vi "Oxford-1820-Main_.vi"() -> ()   [LabVIEW 2016]
uses:
  <instrlib>/Mercury iXX/Public/Controls/Unit String.ctl
  <instrlib>/Mercury iXX/Public/Libraries/Temperature/Controls/Temperature Device (Read).ctl
  <instrlib>/Mercury iXX/Public/Controls/Manufacturing Data.ctl
  <instrlib>/Mercury iXX/Public/Libraries/Temperature/Controls/Temperature Sensor Type.ctl
  <instrlib>/Mercury iXX/Public/Libraries/Temperature/Controls/Excitation Cluster.ctl
  <instrlib>/Mercury iXX/Public/Libraries/Temperature/Controls/Excitation Type.ctl
  <instrlib>/Mercury iXX/Public/Libraries/Temperature/Controls/Calibration Cluster.ctl
  <instrlib>/Mercury iXX/Public/Libraries/Temperature/Controls/Calibration Interpolation.ctl
  <instrlib>/Mercury iXX/Public/Libraries/Temperature/Controls/Loop Cluster.ctl
  <instrlib>/Mercury iXX/Public/Libraries/Temperature/Controls/Temperature Signals Cluster.ctl
  <instrlib>/Mercury iXX/Public/Libraries/Heater/Controls/Heater Device (Read).ctl
  <instrlib>/Mercury iXX/Public/Libraries/Heater/Controls/Heater Signals Cluster.ctl
  <instrlib>/Mercury iXX/Public/Libraries/Level Meter/Controls/Level Meter (Read).ctl
  <instrlib>/Mercury iXX/Public/Libraries/Level Meter/Controls/Nitrogen Configuration.ctl
  <instrlib>/Mercury iXX/Public/Libraries/Level Meter/Controls/Frequency Configuration.ctl
  <instrlib>/Mercury iXX/Public/Libraries/Level Meter/Controls/Signals.ctl
  <instrlib>/Mercury iXX/Public/Libraries/Level Meter/Controls/Helium Configuration.ctl
  <instrlib>/Mercury iXX/Public/Libraries/Level Meter/Controls/Resistance Configuration.ctl
  <instrlib>/Mercury iXX/Public/Libraries/Level Meter/Controls/Pre-Pulse.ctl
  <instrlib>/Mercury iXX/Public/Libraries/Level Meter/Controls/Pulse.ctl
  <instrlib>/Mercury iXX/Public/Libraries/Auxiliary/Controls/AUX Device (Read).ctl
  <instrlib>/Mercury iXX/Public/Libraries/Auxiliary/Controls/AUX Signals (Read).ctl
  <instrlib>/Mercury iXX/Public/Libraries/Magnet/Controls/Device (Read).ctl
  <instrlib>/Mercury iXX/Public/Libraries/Magnet/Controls/Signals (Read).ctl
  <instrlib>/Mercury iXX/Public/Libraries/Magnet/Controls/Identifier.ctl
  <instrlib>/Mercury iXX/Public/Libraries/Pressure/Controls/Pressure Device (Read).ctl
  <instrlib>/Mercury iXX/Public/Libraries/Pressure/Controls/Pressure Sensor Type.ctl
  <instrlib>/Mercury iXX/Public/Libraries/Pressure/Controls/Calibration Cluster.ctl
  <instrlib>/Mercury iXX/Public/Libraries/Pressure/Controls/Calibration Interpolation.ctl
  <instrlib>/Mercury iXX/Public/Libraries/Pressure/Controls/Loop Cluster.ctl
  <instrlib>/Mercury iXX/Public/Libraries/Pressure/Controls/Pressure Signals Cluster.ctl
  <instrlib>/Mercury iXX/Mercury iXX.lvlib
  <instrlib>/Mercury iXX/Public/Controls/Comms Transport Layer.ctl
  <instrlib>/Mercury iXX/Public/Libraries/Pressure/Open/Open Pressure Device.vi
  <instrlib>/Mercury iXX/Public/Libraries/Pressure.lvlib
  <instrlib>/Mercury iXX/Public/Libraries/Pressure/Configuration/Read/Pressure Device (Read).vi
  <instrlib>/Mercury iXX/Public/Libraries/System/Read/Display Automatic Dimming (Read).vi
  <instrlib>/Mercury iXX/Public/Libraries/System.lvlib
  <instrlib>/Mercury iXX/Public/Libraries/System/Read/Display Automatic Dimming Time (Read).vi
  <instrlib>/Mercury iXX/Public/Libraries/System/Read/Display Brightness (Read).vi
  <instrlib>/Mercury iXX/Public/Libraries/System/Read/Mode (Read).vi
  <instrlib>/Mercury iXX/Public/Libraries/System/Read/Serial Number (Read).vi
  <instrlib>/Mercury iXX/Public/Libraries/System/Read/FVer (Read).vi
  <instrlib>/Mercury iXX/Public/Libraries/System/Read/HVer (Read).vi
  <instrlib>/Mercury iXX/Public/Libraries/System/Set/DateTime (Set).vi
  <instrlib>/Mercury iXX/Public/Libraries/Control Loop/Configuration/Read/Control Loop (Read).vi
  <instrlib>/Mercury iXX/Public/Libraries/Control Loop.lvlib
  <instrlib>/Mercury iXX/Public/Libraries/Temperature/Signals/Read/Temperature (Read).vi
  <instrlib>/Mercury iXX/Public/Libraries/Temperature.lvlib
  <instrlib>/Mercury iXX/Public/Libraries/Temperature/Configuration/Read/Calibration Cold Limit (Read).vi
  <instrlib>/Mercury iXX/Public/Libraries/Temperature/Configuration/Read/Calibration Hot Limit (Read).vi
  <instrlib>/Mercury iXX/Public/Libraries/Temperature/Configuration/Read/Excitation Type (Read).vi
  <instrlib>/Mercury iXX/Public/Libraries/Temperature/Configuration/Read/Temperature Sensor (Read).vi
  <instrlib>/Mercury iXX/Public/Libraries/Temperature/Configuration/Read/Temperature Device (Read).vi
  <instrlib>/Mercury iXX/Public/Libraries/Temperature/Configuration/Read/Nickname (Read).vi
  <instrlib>/Mercury iXX/Public/Libraries/Temperature/Configuration/Read/Excitation Magnitude (Read).vi
  <instrlib>/Mercury iXX/Public/Libraries/Temperature/Configuration/Read/Serial Number (Read).vi
  <instrlib>/Mercury iXX/Public/Libraries/System/Read/Catalogue (Read).vi
  <instrlib>/Mercury iXX/Public/Libraries/System/Read/Flash Space (Read).vi
  <instrlib>/Mercury iXX/Public/Libraries/System/Read/DateTime (Read).vi
  <instrlib>/Mercury iXX/Public/Libraries/System/Read/Time (Read).vi
  <instrlib>/Mercury iXX/Public/Libraries/System/Read/Date (Read).vi
  <instrlib>/Mercury iXX/Public/Libraries/System/Open/Open System.vi
  <instrlib>/Mercury iXX/Public/Libraries/Temperature/Open/Open Temperature Device.vi
  <instrlib>/Mercury iXX/Public/Libraries/Auxiliary/Open/Open Auxiliary Device.vi
  <instrlib>/Mercury iXX/Public/Libraries/Auxiliary.lvlib
  <instrlib>/Mercury iXX/Public/Libraries/Auxiliary/Signals/Read/Percent Open (Read).vi
  <instrlib>/Mercury iXX/Public/Libraries/Magnet/Open/Open Magnet Device.vi
  <instrlib>/Mercury iXX/Public/Libraries/Magnet.lvlib
  <instrlib>/Mercury iXX/Public/Libraries/Magnet/Configuration/Read/PSU Action Status (Read).vi
  <instrlib>/Mercury iXX/Public/Libraries/Magnet/Configuration/Read/Magnet Device (Read).vi
  <instrlib>/Mercury iXX/Public/Libraries/Temperature/Signals/Read/Voltage (Read).vi
  <instrlib>/Mercury iXX/Private/Controls/Query Dynamic Reference.ctl
  <instrlib>/Mercury iXX/Public/Controls/Mercury Reference.ctl
  <instrlib>/Mercury iXX/Public/Libraries/Level Meter/Open/Open Level Meter Device.vi
  <instrlib>/Mercury iXX/Public/Libraries/Level Meter.lvlib
  <instrlib>/Mercury iXX/Public/Libraries/Level Meter/Signals/Read/Probe Level Nitrogen (Read).vi
  <instrlib>/Mercury iXX/Public/Libraries/Level Meter/Signals/Read/Probe Level Helium (Read).vi
  <instrlib>/Mercury iXX/Public/Libraries/Magnet/Signals/Read/Switch Heater Status (Read).vi
  <instrlib>/Mercury iXX/Public/Libraries/Magnet/Signals/Read/Current (Read).vi
  <instrlib>/Mercury iXX/Public/Libraries/Magnet/Configuration/Set/PSU Action Status (Set).vi
  <instrlib>/Mercury iXX/Public/Libraries/Magnet/Controls/PSU Actions.ctl
  SMOs/Instrument.Oxford1820/Instrument.Oxford1820.lvclass
  <instrlib>/Mercury iXX/Public/Controls/ISOBus Address.ctl
  <instrlib>/Mercury iXX/Public/Libraries/Lambda/Configuration/Set/Lambda Percentage Flow (Set).vi
  <instrlib>/Mercury iXX/Public/Libraries/Lambda.lvlib
  <instrlib>/Mercury iXX/Public/Libraries/Lambda/Open/Open Lambda Device.vi
  <instrlib>/Mercury iXX/Public/Controls/Response String.ctl
  <instrlib>/Mercury iXX/Public/Libraries/Temperature/Signals/Read/Resistance (Read).vi
  <instrlib>/Mercury iXX/Public/Libraries/Magnet/Controls/Switch Heater.ctl
  <instrlib>/Mercury iXX/Public/Libraries/Heater/Configuration/Read/Serial Number (Read).vi
  <instrlib>/Mercury iXX/Public/Libraries/Heater.lvlib
  <instrlib>/Mercury iXX/Public/Libraries/Pressure/Configuration/Read/Nickname (Read).vi
  <instrlib>/Mercury iXX/Public/Libraries/Level Meter/Configuration/Set/Pulse Slow-Fast (Set).vi
  <instrlib>/Mercury iXX/Public/Libraries/Magnet/Signals/Set/Target Field Rate (Set).vi
  <instrlib>/Mercury iXX/Public/Libraries/Auxiliary/Configuration/Read/Stepper Speed (Read).vi
  <instrlib>/Mercury iXX/Public/Libraries/Heater/Configuration/Read/Nickname (Read).vi
  <instrlib>/Mercury iXX/Public/Libraries/Auxiliary/Signals/Read/Position (Read).vi
  <instrlib>/Mercury iXX/Public/Libraries/Pressure/Signals/Read/Current (Read).vi
  <instrlib>/Mercury iXX/Public/Libraries/Auxiliary/Configuration/Read/Temperature Error Voltage Sensitivity (Read).vi
  <instrlib>/Mercury iXX/Public/Libraries/Heater/Signals/Read/Voltage (Read).vi
  <instrlib>/Mercury iXX/Public/Libraries/Heater/Configuration/Read/Maximum Power (Read).vi
  <instrlib>/Mercury iXX/Public/Libraries/Auxiliary/Configuration/Read/Temperature Error Sensitivity (Read).vi
  <instrlib>/Mercury iXX/Public/Libraries/Auxiliary/Configuration/Read/Aux Device (Read).vi
  <instrlib>/Mercury iXX/Public/Libraries/Heater/Open/Open Heater Device.vi
  <instrlib>/Mercury iXX/Public/Libraries/Heater/Signals/Read/Current (Read).vi
  <userlib>/_OpenG.lib/error/error.llb/Filter Error Codes (Array)__ogtk.vi
  <instrlib>/Mercury iXX/Public/Libraries/Lambda/Configuration/Set/Lambda Flow Auto (Set).vi
  <instrlib>/Mercury iXX/Public/Libraries/Heater/Configuration/Read/Heater Device (Read).vi
  <instrlib>/Mercury iXX/Public/Libraries/Auxiliary/Configuration/Read/Valve Gearing (Read).vi
  <instrlib>/Mercury iXX/Public/Libraries/Auxiliary/Configuration/Read/Serial Number (Read).vi
  <instrlib>/Mercury iXX/Public/Libraries/Heater/Configuration/Read/Voltage Limit (Read).vi
  <instrlib>/Mercury iXX/Public/Libraries/Heater/Configuration/Read/Nominal Resistance (Read).vi
  <instrlib>/Mercury iXX/Public/Libraries/Pressure/Signals/Read/Voltage (Read).vi
  <instrlib>/Mercury iXX/Public/Libraries/Magnet/Signals/Set/Target Field (Set).vi
  <instrlib>/Mercury iXX/Public/Libraries/Magnet/Signals/Read/Persistant Current (Read).vi
  <instrlib>/Mercury iXX/Public/Libraries/Auxiliary/Configuration/Read/Minimum Gas Flow (Read).vi
  <instrlib>/Mercury iXX/Public/Libraries/Heater/Signals/Read/Power (Read).vi
  <instrlib>/Mercury iXX/Public/Libraries/Auxiliary/Configuration/Read/Gas Flow Scaling (Read).vi
  <instrlib>/Mercury iXX/Public/Libraries/Magnet/Signals/Set/Switch Heater Status (Set).vi
  <instrlib>/Mercury iXX/Public/Libraries/Level Meter/Configuration/Read/Nitrogen Freq at 100 (Read).vi
  <instrlib>/Mercury iXX/Public/Libraries/Magnet/Configuration/Read/Serial Number (Read).vi
  <instrlib>/Mercury iXX/Public/Libraries/Magnet/Signals/Read/Field (Read).vi
  <instrlib>/Mercury iXX/Public/Libraries/Level Meter/Configuration/Read/Helium Pulse Mag (Read).vi
  <instrlib>/Mercury iXX/Public/Libraries/Level Meter/Configuration/Read/Helium Probe Resistance (Read).vi
  <instrlib>/Mercury iXX/Public/Libraries/Magnet/Signals/Read/Voltage (Read).vi
  <instrlib>/Mercury iXX/Public/Libraries/Magnet/Configuration/Read/Current to Field Factor (Read).vi
  <instrlib>/Mercury iXX/Public/Libraries/Magnet/Signals/Read/Target Field (Read).vi
  <instrlib>/Mercury iXX/Public/Libraries/Magnet/Configuration/Read/Bipolar Output (Read).vi
  <instrlib>/Mercury iXX/Public/Libraries/Magnet/Configuration/Read/Current Limit (Read).vi
  <instrlib>/Mercury iXX/Public/Libraries/Magnet/Signals/Read/Persistant Field (Read).vi
  <instrlib>/Mercury iXX/Public/Libraries/Level Meter/Configuration/Read/Serial Number (Read).vi
  <instrlib>/Mercury iXX/Public/Libraries/Magnet/Signals/Read/Current Rate (Read).vi
  <instrlib>/Mercury iXX/Public/Libraries/Magnet/Signals/Read/Target Field Rate (Read).vi
  <instrlib>/Mercury iXX/Public/Libraries/Level Meter/Configuration/Read/Level Meter Device (Read).vi
  <instrlib>/Mercury iXX/Public/Libraries/Level Meter/Signals/Read/Probe Resistance Helium (Read).vi
  <instrlib>/Mercury iXX/Public/Libraries/Magnet/Configuration/Read/Output Configuration (Read).vi
  <instrlib>/Mercury iXX/Public/Libraries/Level Meter/Configuration/Read/Nitrogen Pulse Count Period (Read).vi
  <instrlib>/Mercury iXX/Public/Libraries/Magnet/Configuration/Read/Software Voltage Limit (Read).vi
  <instrlib>/Mercury iXX/Public/Libraries/Level Meter/Configuration/Read/Helium Pulse Duration (Read).vi
  <instrlib>/Mercury iXX/Public/Libraries/Level Meter/Signals/Read/Probe Count Nitrogen (Read).vi
  <instrlib>/Mercury iXX/Public/Libraries/Magnet/Configuration/Read/Switch Present (Read).vi
panel:
  in  "Tab Control 6":enum32{"Page 1", "Page 2"}(tab)
  in  "Tab Control 5":enum32{"Page 1", "Page 2"}(tab)
  in  "Open Needle Valve":bool
  in  "Close Needle Valve":bool
  in  "Lambda":bool
  out "LPF NV (%)":dbl format="%_6g"
  out "LPF Pressure":dbl format="%_5f mB"
  out "Magnet Field (T) 2":dbl(knob) caption="Voltage (V)" scale=-20.0..20.0
  out "Voltage (V) 2":dbl(knob)=-0.0003 caption="Voltage (V)" scale=-10.0..10.0
  out "Current (A)":dbl(knob)=0.0006 scale=-180.0..180.0
  in  "Tab Control 4":enum32{"Page 1", "Page 2"}(tab)
  out "N2 LEVEL":dbl=61.3025 format="%.0f %"
  out "He LVL Chart":dbl(slide)=52.0833 scale=0.0..100.0
  out "N2 LVL Chart":dbl(slide)=61.3025 scale=0.0..100.0
  out "He LEVEL 3":dbl=61.3025 format="%.0f %"
  in  "Fast/Slow Fill":bool
  in  "Tab Control 3":enum32{"Page 1", "Page 2"}(tab)
  out "Magnet T":dbl=3.8705 format="%_2f K"
  out "Magnet R":dbl=3.8705 format="%_3f ohms"
  out "LPF R":dbl=4.2075 format="%_3f ohms"
  out "Voltage (V)":dbl=-0.0003 format="%.5f"
  out "LPF T":dbl=4.2075 format="%_2f K"
  out "Current (A)":dbl=0.0006 format="%.5f"
  out "Magnet Status 2":string
  in  "Tab Control 2":enum32{"Page 1", "Page 2"}(tab)
  in  "Hold":bool
  in  "To Set":bool
  in  "Send to IPS":bool
  out "Power Supply Field (T)":dbl=0.0001 format="%#.5f"
  in  "Target Field (T) 2":dbl format="%#.5f"
  out "Target Field (T)":dbl format="%#.5f"
  in  "Target Rate (T/min)":dbl=0.1 format="%.5f"
  out "Target  Rate (T/min)":dbl=1.0 format="%.5f"
  out "Magnet Field (T)":dbl format="%.5f"
  out "He LEVEL":dbl=52.0833 format="%.0f %"
  in  "PS Heat":bool
  out "Switch Time":string="11:11:48"
  in  "To Zero":bool
  in  "Clamp":bool
  in  "Toolbar":enum32{"Page 1", "Page 2"}(tab)
  in  "Start 2":bool
  in  "Stop 2":bool
  in  "Window Minimize":bool
  out "ETA":string
  out "Magnet Status 3":string="Clamped"
  in  "Remote Mode":bool
  out "Sentinel":bool=TRUE
  in  "Window Maximize":bool
  out "SWITCH HEATER":bool
  out "LPF ON":timestamp
  in  "Tab Control":T1(tab)
  in  "Mercury Functions":T2(tab)=enum."Temperature"
  out "time stamp":timestamp=timestamp(3543841780 s since 1904-01-01)
  out "Free Space":i32=166384 caption="Free Space (KB)"
  out "Set Date Response":string="VALID"
  out "String":string="NORM" caption="User Mode"
  out "Date":string="2016:04:18"
  out "Time":string="11:29:40"
  out "Hardware Version":string="65"
  out "Firmware Version":string="2.2.6.20"
  out "Serial Number":string="154650110"
  out "ITC Devices":string[](array[string])=["DB4.G1:AUX", "DB8.P1:PRES", "MB0.H1:HTR", "MB1.T1:TEMP"]
  out "S/W Version(s)":string[](array[string])=["2.2.6.20\n"]
  out "Serial Number(s)":string[](array[string])=["154650110"]
  out "# of Instruments":i32=1
  out "Automatic Dimming":string="OFF"
  out "Dimming Time":string="5"
  out "Display Brightness":string="100"
  in  "ITC IP Address":string="130.49.180.101"
  out "Excitation Magnitude":dbl=5.0
  out "Sensor Type":string="NTC"
  out "Excitation Type":string="UNIP"
  out "Hot Limit":dbl=1000.0
  out "H Unit":T3="K"
  out "Cold Limit":dbl=1000.0
  out "C Unit":T3="K"
  out "Unit":T3
  out "Voltage":dbl=0.005
  out "V Unit":T3="V"
  out "Temperature":dbl=4.2075
  out "T Unit":T3="K"
  out "Temperature Device Settings":T4={"Manufacturing"={"Hardware Version"="65", "Firmware Version"="2.2", "Serial Number"="154650110"}, "Temperature Sensor Type"="NTC", "Excitation"={"Excitation Type"="UNIP", "Magnitude"="5.00"}, "Calibration"={"Filename"="59543_iTC-lambda.dat", "Interpolation"="LIN", "Scaling Factor"="1", "Offset Factor"="0", "Hot Limit"="1000.00K", "Cold Limit"="1000.00K", "Last Calibration"="", "Reference"="Internal"}, "Control Loop"={"Heater"="", "Auxiliary"="", "Heater Auto"="", "Percentage Heat"="", "Temperature Set Point"="", "PID Auto (from file)"="", "P Value"="", "I Value"="", "D Value"="", "Auto PID Table Filename"="", "Flow Auto"="", "Target Heater Table"="", "Sweep mode"="", "Sweep Table Filename"="", "Percentage Flow"=""}, "Temperature Signals"={"Voltage"="5.0000mV", "Current"="3.9694µA", "Power"="0.0199µW", "Resistance"="1259.6510R", "Temperature"="4.2075K", "Sensitivity"="299.3801R/K", "Reference"="N/A"}, "Nickname"="Mag_AB_MB1", "Status"="0"}
  out "Temp S/N":string="154650110"
  out "T Nickname":string="Mag_AB_MB1"
  out "T Loop Details":T11
  out "Heater Device Settings":T13={"Manufacturing"={"Hardware Version"="65", "Firmware Version"="2.3", "Serial Number"="154650110"}, "Nickname"="MB0.H1", "Voltage Limit"="1", "Nominal Resistance"="10", "Maximum Power"="0.1000", "Heater Signals"={"Voltage"="0.0507V", "Current"="-0.0000A", "Power"="0.0000W"}, "Status"="2"}
  out "Htr C Unit":T3="A"
  out "Htr P Unit":T3="W"
  out "Htr V Unit":T3="V"
  out "Htr Current":dbl=-0.0
  out "Htr Power":dbl
  out "Htr Voltage":dbl=0.0507
  out "Power Unit":T3
  out "Volt Unit":T3
  out "Res Unit":T3
  out "Maximum Power":dbl=0.1
  out "Htr Resistance":dbl=10.0
  out "Htr Voltage Limit":dbl=1.0
  out "Htr S/N":string="154650110"
  out "Htr Nickname":string="MB0.H1"
  out "Pressure Device":T15={"Manufacturing"={"Hardware Version"="3", "Firmware Version"="1.10", "Serial Number"="151150091"}, "Temperature Sensor Type"="RAT", "Calibration"={"Filename"="Lambda pressure control_10V ratiometric.dat", "Interpolation"="LIN", "Scaling Factor"="1", "Offset Factor"="-0.0004", "High Limit"="1000.00K", "Low Limit"="1000.00K", "Last Calibration"=""}, "Control Loop"={"Heater"="None", "Auxiliary"="None", "Heater Auto"="", "Percentage Heat"="", "Pressure Set Point"="", "PID Auto (from file)"="", "P Value"="", "I Value"="", "D Value"="1.0", "Auto PID Table Filename"="", "Flow Auto"="", "Target Heater Table"="", "Sweep mode"="", "Sweep Table Filename"="", "Percentage Flow"=""}, "Pressure Signals"={"Voltage"="-0.0822mV", "Current"="-0.0000A", "Power"="0.0000W", "Pressure"="0.0000mB"}, "Nickname"="Lam_P_DB8", "Status"="0"}
  out "Nickname":string="Lam_P_DB8"
  out "Current":dbl=-0.0
  out "Voltage":dbl=-8.219999999999999e-05
  out "Auxiliary Device Details":T21={"Manufacturing"={"Hardware Version"="65", "Firmware Version"="3.1", "Serial Number"="154650084"}, "Min Flow"=0.0, "Scaling Factor"=50.0, "Temp Err"=9.0, "Temp V Err"=11.0, "Gear"=2, "Speed"=2, "Signals"={"Position"=0.0, "% Open"=0.0, "I0"="ON", "I1"="OFF", "I2"="OFF", "I3"="OFF", "O0"="OFF", "O1"="OFF", "O2"="OFF", "O3"="OFF"}, "Nickname"="DB4.G1", "Status"="0"} {"Signals"."% Open" min=0.0 max=100.0 step=0.1 format="%.4f"; "Signals"."Position" max=20.0 step=1.0 format="%.4f"; "Speed" max=7 step=1; "Gear" max=7 step=1; "Temp V Err" min=0.0 max=20.0 step=0.1; "Temp Err" min=0.0 max=20.0 step=0.1; "Scaling Factor" min=0.0 max=99.0 step=0.1; "Min Flow" min=0.0 max=20.0 step=0.1}
  out "Aux S/N":string="154650084"
  out "Min Flow":dbl caption="Minimum Gas Flow" format="%#.1f"
  out "Scaling Factor":dbl=50.0 caption="Gas Flow Scaling Factor" format="%#.1f"
  out "Temp Err":dbl=9.0 caption="Temperature Error Sensitivity" format="%#.1f"
  out "Temp V Err":dbl=11.0 caption="Temperature Voltage Error Sensitivity" format="%#.1f"
  out "Gear":u32=2 caption="Valve Gearing"
  out "Speed":u32=2 caption="Stepper Speed"
  out "Unit 2":T3
  out "Unit 3":T3
  out "Unit 4":T3
  out "Unit 5":T3
  out "Unit 6":T3
  out "Unit 7":T3
  out "Position":u32
  out "% Open":dbl caption="Percentage Open (%)"
  out "Unit":T3
  out "Unit":T3="%"
  out "time stamp 2":timestamp=timestamp(3543841781 s since 1904-01-01)
  out "Free Space 2":i32=166316 caption="Free Space (KB)"
  out "Set Date Response 2":string="VALID"
  out "String 2":string="NORM" caption="User Mode"
  out "Date 2":string="2016:04:18"
  out "Time 2":string="11:29:45"
  out "Hardware Version 2":string="65"
  out "Firmware Version 2":string="2.2.6.20"
  out "Serial Number 2":string="153350063"
  out "IPS Devices":string[](array[string])=["DB3.L1:LVL", "GRPX:PSU", "GRPY:PSU", "GRPZ:PSU", "MB1.T1:TEMP", "PSU.M1:PSU", "PSU.M2:PSU", "PSU.M3:PSU"]
  out "S/W Version(s) 2":string[](array[string])=["2.2.6.20\n"]
  out "Serial Number(s) 2":string[](array[string])=["153350063"]
  out "# of Instruments 2":i32=1
  out "Automatic Dimming 2":string="OFF"
  out "Dimming Time 2":string="5"
  out "Display Brightness 2":string="100"
  in  "IPS IP Address":string="130.49.180.102"
  out "LVL Device DetailSettings":T23={"Manufacturing"={"Hardware Version"="65", "Firmware Version"="2.2", "Serial Number"="152450013"}, "Nitrogen Configuration"={"Frequency Configuration"={"Freq 0%"=0.0, "Freq 100%"=0.0}, "Pulse Period"=0.0}, "Signals"={"Helium Signals"={"Resistance"=75.5626, "Level"=52.0833}, "Nitrogen Signals"={"Count"=8800.0, "Freq"=487361.0, "Level"=61.3445}}, "Nickname"="DB3.L1", "Status"="0", "Helium Configuration"={"Resistance Configuration"={"Res 0%"=0.0, "Res 100%"=0.0}, "Pre-Pulse"={"Magnitude"=0.0, "Duration"=0.0}, "Pulse"={"Magnitude"=0.0, "Duration"=0.0, "Delay"=0.0}}}
  out "LVL S/N":string="152450013"
  out "LVL P Magnitude":dbl=125.0 caption="Pulse Magnitude (mA)"
  out "LVL P Duration":dbl=5.0 caption="Pulse Duration (s)"
  out "N Freq 100%":dbl=7880.0 caption="Frequency at 100% (Hz)"
  out "N Pulse Period":dbl=1000.0 caption="Pulse Period (ms)"
  out "He Res Config":T28={"Res 0%"=149.0, "Res 100%"=8.0}
  out "He Resistance":dbl=75.5626 caption="Resistance (Ohms)"
  out "He Level":dbl=52.0833 caption="Helium Level (%)"
  out "N Counter":u32 caption="Counter"
  out "N Level":dbl=61.3445 caption="Nitrogen Level (%)"
  out "Excitation Magnitude 2":dbl=5.0
  out "Sensor Type 2":string="NTC"
  out "Excitation Type 2":string="UNIP"
  out "Hot Limit 2":dbl=1000.0
  out "H Unit 2":T3="K"
  out "Cold Limit 2":dbl=1000.0
  out "C Unit 2":T3="K"
  out "Unit 12":T3
  out "Voltage 2":dbl=0.005
  out "V Unit 2":T3="V"
  out "Temperature 2":dbl=3.8706
  out "T Unit 2":T3="K"
  out "Temperature Device Settings 2":T4={"Manufacturing"={"Hardware Version"="65", "Firmware Version"="2.2", "Serial Number"="153350063"}, "Temperature Sensor Type"="NTC", "Excitation"={"Excitation Type"="UNIP", "Magnitude"="5.00"}, "Calibration"={"Filename"="Bob.dat", "Interpolation"="LIN", "Scaling Factor"="1", "Offset Factor"="0", "Hot Limit"="1000.00K", "Cold Limit"="1000.00K", "Last Calibration"="", "Reference"="Internal"}, "Control Loop"={"Heater"="", "Auxiliary"="", "Heater Auto"="", "Percentage Heat"="", "Temperature Set Point"="", "PID Auto (from file)"="", "P Value"="", "I Value"="", "D Value"="", "Auto PID Table Filename"="", "Flow Auto"="", "Target Heater Table"="", "Sweep mode"="", "Sweep Table Filename"="", "Percentage Flow"=""}, "Temperature Signals"={"Voltage"="5.0000mV", "Current"="3.5897µA", "Power"="0.0179µW", "Resistance"="1392.8897R", "Temperature"="3.8706K", "Sensitivity"="359.8580R/K", "Reference"="N/A"}, "Nickname"="MB1.T1", "Status"="0"}
  out "Temp S/N 2":string="153350063"
  out "T Nickname 2":string="MB1.T1"
  out "T Loop Details 2":T11
  out "Magnet Device Details":T31={"Manufacturing"={"Hardware Version"="NOT_FOUND", "Firmware Version"="NOT_FOUND", "Serial Number"="NOT_FOUND"}, "Nickname"="GRPZ", "Bipolar Output"="ON", "String"="PARA", "Current Limit"=174.0, "AtoB"=8.688, "Inductance"=39.406, "Switch Present"="PSU.M1", "Swh Htr Current"=86.0, "SW VLIM"=9.0, "V Trans Time"=1000.0, "Magnet PSU Signals"={"Voltage"=-0.0002, "Current"=0.0002, "Current Rate"=100.0, "Field"=0.0001, "Field Rate"=11.5101, "Persistant Current"=0.0003, "Persistant Field"=0.0, "Target Current"=0.0, "Target Field"=0.0, "Target Current Rate"=8.688, "Target Field Rate"=1.0, "Switch Heater Status (SWHT)"="OFF", "Switch Heater Status (SWHN)"="OFF"}, "PSU Action"="CLMP", "Status"="40000000", "Level Limit"=0.0, "Temperature Limit"=999.0} {"Temperature Limit" format="%#.1f"; "Level Limit" format="%#.1f"; "V Trans Time" format="%#.1f"; "SW VLIM" format="%#.1f"; "Swh Htr Current" format="%#.1f"; "Inductance" format="%#.1f"; "AtoB" format="%#.1f"; "Current Limit" format="%#.1f"}
  out "Mag S/N":string="NOT_FOUND"
  out "Bipolar Output":string="ON"
  out "Out Config":string="PARA" caption="Output Configuration"
  out "Current Limit":dbl=174.0 caption="Current Limit (A)" format="%#.1f"
  out "AtoB":dbl=8.688 caption="Current Field Factor (A/T)" format="%#.1f"
  out "Switch Present":string="PSU.M1"
  out "SW VLIM":dbl=9.0 caption="Software Voltage Limit (V)" format="%#.1f"
  out "Unit 8":T3
  out "Unit 9":T3
  out "Unit 10":T3
  out "Current Rate":dbl=100.0
  out "PSU Act Stat":string="CLMP" caption="PSU Action Status"
  out "Unit 11":T3="A/min"
  in  "Device Identifier":T33="GRPZ"
  out "Error List":T34(array[cluster])
  out "LPF on (s)":i32=5373
  # "Magnet (T)"
  # "Voltage (V)"
  # "Current (A)"
  # "Slow Rates\nCurrent Range (A)     Field Range (T)   Rate (T/min)\n0       -- 100        0    -- 11.5      0.91\n100     -- 150        11.5 -- 17.2      0.23\n150     -- 155.467    17.2 -- 18        0.11\n155.567 -- 172.471    18   -- 20        0.11\n\nFast Rates\nCurrent Range (A)     Field Range (T)   Rate (T/min)\n0       -- 155.467    0    -- 18        1.0\n155.567 -- 172.471    18   -- 20        0.25"
  # "Helium"
  # "Nitrogen"
  # "v17/02/01"
  # "ITC: 101\nIPS: 102\nIPS VR: 67"
  # "ITC: 101\nIPS: 102\nIPS VR: 67"
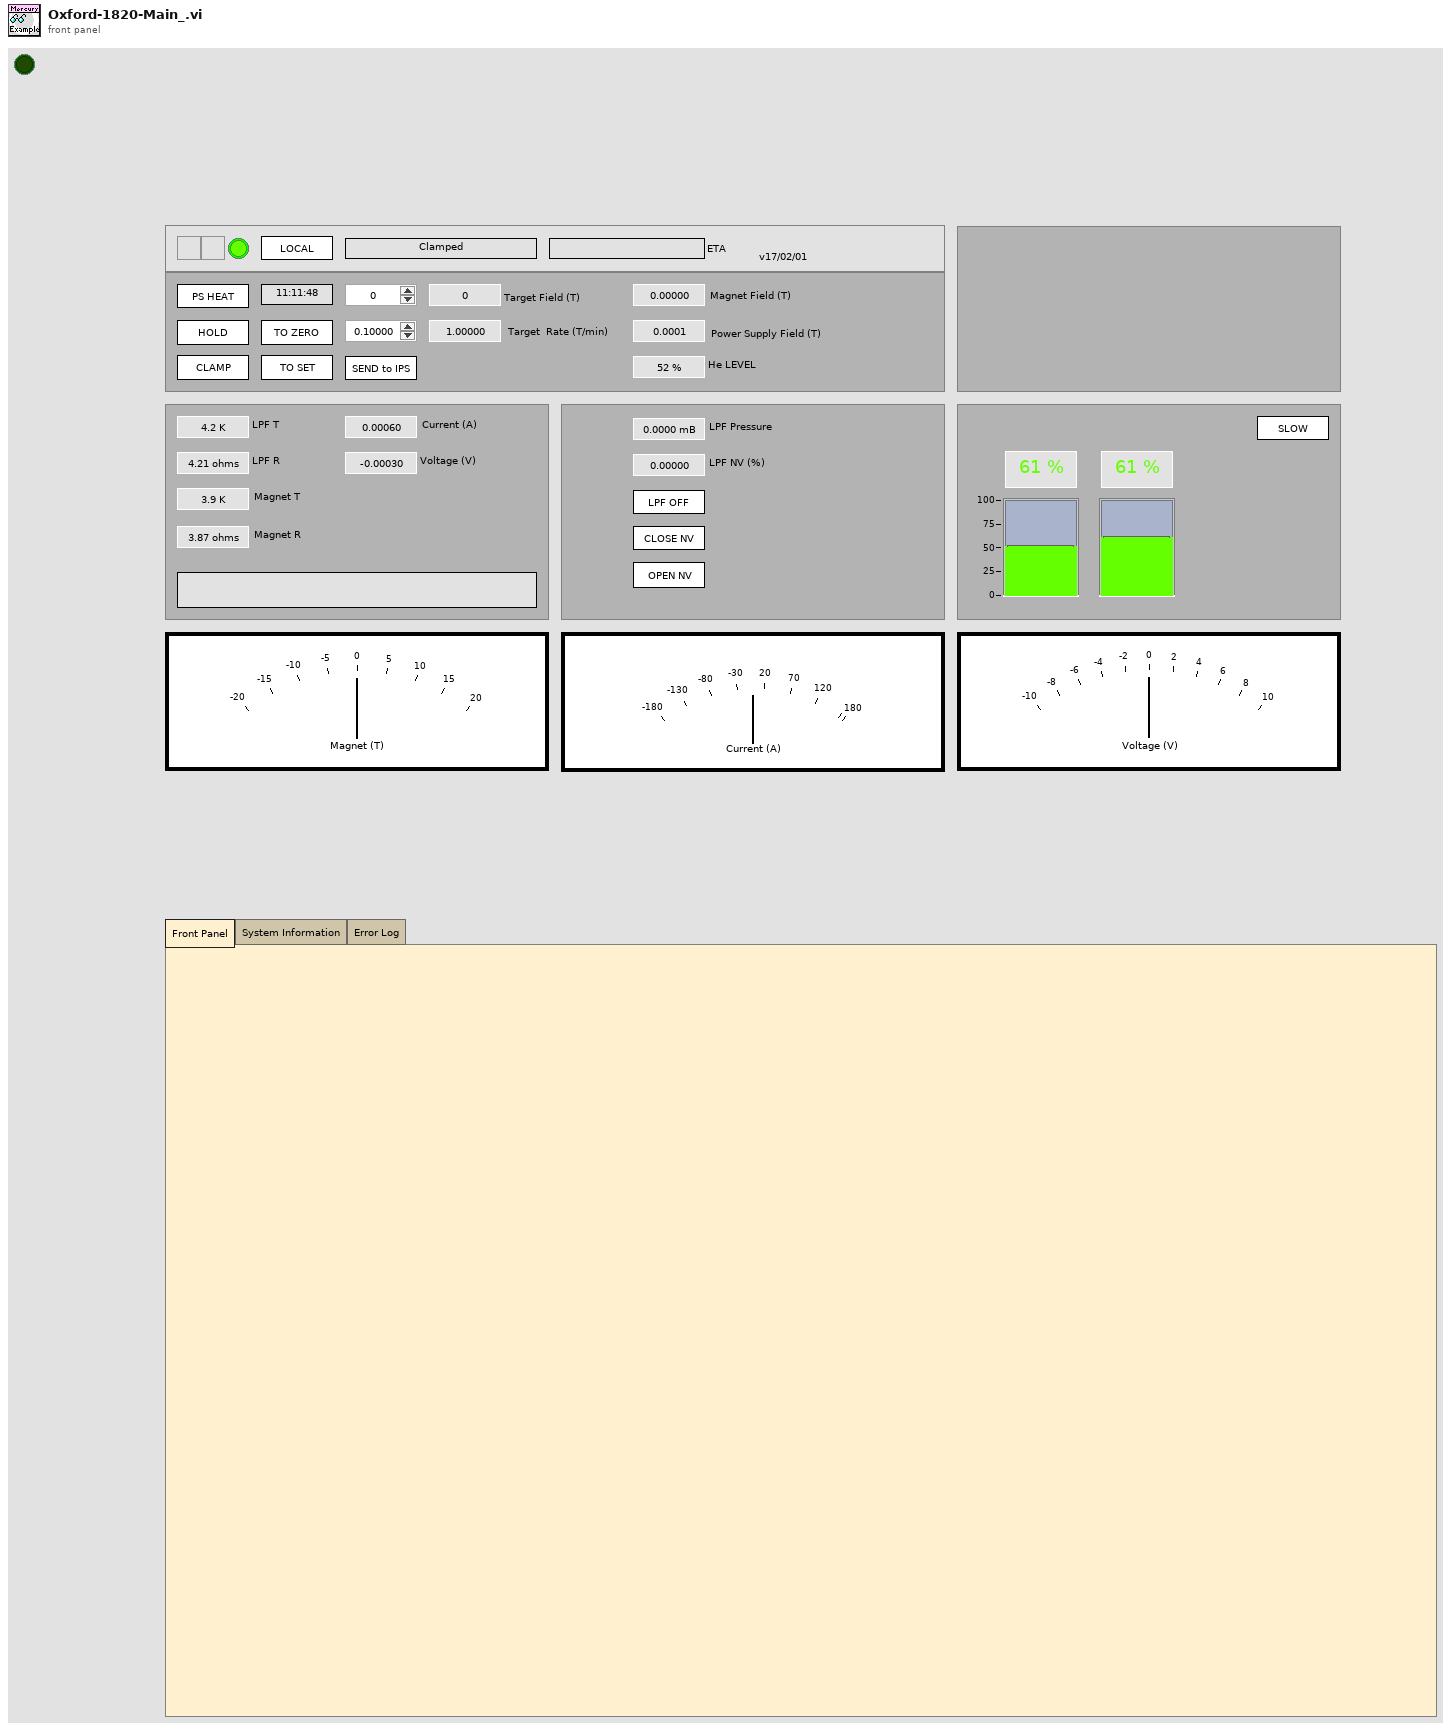
[diagram p1: front panel]
types:
  T1 = enum32{"Front Panel", "System Information", "Error Log"}
  T2 = enum32{"System: ITC", "Temperature", "Heater", "Pressure", "Auxiliary", "System: IPS", "Level Meter", "Temperature 2", "Magnet"}
  T3 = typedef "Mercury iXX.lvlib/Unit String.ctl" = string
  T4 = typedef "Mercury iXX.lvlib/Temperature.lvlib/Temperature Device (Read).ctl" = cluster{"Manufacturing":T5, "Temperature Sensor Type":T6, "Excitation":T7, "Calibration":T9, "Control Loop":T11, "Temperature Signals":T12, "Nickname":string, "Status":string}
  T5 = typedef "Mercury iXX.lvlib/Manufacturing Data.ctl" = cluster{"Hardware Version":string, "Firmware Version":string, "Serial Number":string}
  T6 = typedef "Mercury iXX.lvlib/Temperature.lvlib/Temperature Sensor Type.ctl" = string
  T7 = typedef "Mercury iXX.lvlib/Temperature.lvlib/Excitation Cluster.ctl" = cluster{"Excitation Type":T8, "Magnitude":string}
  T8 = typedef "Mercury iXX.lvlib/Temperature.lvlib/Excitation Type.ctl" = string
  T9 = typedef "Mercury iXX.lvlib/Temperature.lvlib/Calibration Cluster.ctl" = cluster{"Filename":string, "Interpolation":T10, "Scaling Factor":string, "Offset Factor":string, "Hot Limit":string, "Cold Limit":string, "Last Calibration":string, "Reference":string}
  T10 = typedef "Mercury iXX.lvlib/Temperature.lvlib/Calibration Interpolation.ctl" = string
  T11 = typedef "Mercury iXX.lvlib/Temperature.lvlib/Loop Cluster.ctl" = cluster{"Heater":string, "Auxiliary":string, "Heater Auto":string, "Percentage Heat":string, "Temperature Set Point":string, "PID Auto (from file)":string, "P Value":string, "I Value":string, "D Value":string, "Auto PID Table Filename":string, "Flow Auto":string, "Target Heater Table":string, "Sweep mode":string, "Sweep Table Filename":string, "Percentage Flow":string}
  T12 = typedef "Mercury iXX.lvlib/Temperature.lvlib/Temperature Signals Cluster.ctl" = cluster{"Voltage":string, "Current":string, "Power":string, "Resistance":string, "Temperature":string, "Sensitivity":string, "Reference":string}
  T13 = typedef "Mercury iXX.lvlib/Heater.lvlib/Heater Device (Read).ctl" = cluster{"Manufacturing":T5, "Nickname":string, "Voltage Limit":string, "Nominal Resistance":string, "Maximum Power":string, "Heater Signals":T14, "Status":string}
  T14 = typedef "Mercury iXX.lvlib/Heater.lvlib/Heater Signals Cluster.ctl" = cluster{"Voltage":string, "Current":string, "Power":string}
  T15 = typedef "Mercury iXX.lvlib/Pressure.lvlib/Pressure Device (Read).ctl" = cluster{"Manufacturing":T5, "Temperature Sensor Type":T16, "Calibration":T17, "Control Loop":T19, "Pressure Signals":T20, "Nickname":string, "Status":string}
  T16 = typedef "Mercury iXX.lvlib/Pressure.lvlib/Pressure Sensor Type.ctl" = string
  T17 = typedef "Mercury iXX.lvlib/Pressure.lvlib/Calibration Cluster.ctl" = cluster{"Filename":string, "Interpolation":T18, "Scaling Factor":string, "Offset Factor":string, "High Limit":string, "Low Limit":string, "Last Calibration":string}
  T18 = typedef "Mercury iXX.lvlib/Pressure.lvlib/Calibration Interpolation.ctl" = string
  T19 = typedef "Mercury iXX.lvlib/Pressure.lvlib/Loop Cluster.ctl" = cluster{"Heater":string, "Auxiliary":string, "Heater Auto":string, "Percentage Heat":string, "Pressure Set Point":string, "PID Auto (from file)":string, "P Value":string, "I Value":string, "D Value":string, "Auto PID Table Filename":string, "Flow Auto":string, "Target Heater Table":string, "Sweep mode":string, "Sweep Table Filename":string, "Percentage Flow":string}
  T20 = typedef "Mercury iXX.lvlib/Pressure.lvlib/Pressure Signals Cluster.ctl" = cluster{"Voltage":string, "Current":string, "Power":string, "Pressure":string}
  T21 = typedef "Mercury iXX.lvlib/Auxiliary.lvlib/AUX Device (Read).ctl" = cluster{"Manufacturing":T5, "Min Flow":dbl, "Scaling Factor":dbl, "Temp Err":dbl, "Temp V Err":dbl, "Gear":u32, "Speed":u32, "Signals":T22, "Nickname":string, "Status":string}
  T22 = typedef "Mercury iXX.lvlib/Auxiliary.lvlib/AUX Signals (Read).ctl" = cluster{"Position":dbl, "% Open":dbl, "I0":string, "I1":string, "I2":string, "I3":string, "O0":string, "O1":string, "O2":string, "O3":string}
  T23 = typedef "Mercury iXX.lvlib/Level Meter.lvlib/Level Meter (Read).ctl" = cluster{"Manufacturing":T5, "Nitrogen Configuration":T24, "Signals":T26, "Nickname":string, "Status":string, "Helium Configuration":T27}
  T24 = typedef "Mercury iXX.lvlib/Level Meter.lvlib/Nitrogen Configuration.ctl" = cluster{"Frequency Configuration":T25, "Pulse Period":dbl}
  T25 = typedef "Mercury iXX.lvlib/Level Meter.lvlib/Frequency Configuration.ctl" = cluster{"Freq 0%":dbl, "Freq 100%":dbl}
  T26 = typedef "Mercury iXX.lvlib/Level Meter.lvlib/Signals.ctl" = cluster{"Helium Signals":cluster{"Resistance":dbl, "Level":dbl}, "Nitrogen Signals":cluster{"Count":dbl, "Freq":dbl, "Level":dbl}}
  T27 = typedef "Mercury iXX.lvlib/Level Meter.lvlib/Helium Configuration.ctl" = cluster{"Resistance Configuration":T28, "Pre-Pulse":T29, "Pulse":T30}
  T28 = typedef "Mercury iXX.lvlib/Level Meter.lvlib/Resistance Configuration.ctl" = cluster{"Res 0%":dbl, "Res 100%":dbl}
  T29 = typedef "Mercury iXX.lvlib/Level Meter.lvlib/Pre-Pulse.ctl" = cluster{"Magnitude":dbl, "Duration":dbl}
  T30 = typedef "Mercury iXX.lvlib/Level Meter.lvlib/Pulse.ctl" = cluster{"Magnitude":dbl, "Duration":dbl, "Delay":dbl}
  T31 = typedef "Mercury iXX.lvlib/Magnet.lvlib/Device (Read).ctl" = cluster{"Manufacturing":T5, "Nickname":string, "Bipolar Output":string, "String":string, "Current Limit":dbl, "AtoB":dbl, "Inductance":dbl, "Switch Present":string, "Swh Htr Current":dbl, "SW VLIM":dbl, "V Trans Time":dbl, "Magnet PSU Signals":T32, "PSU Action":string, "Status":string, "Level Limit":dbl, "Temperature Limit":dbl}
  T32 = typedef "Mercury iXX.lvlib/Magnet.lvlib/Signals (Read).ctl" = cluster{"Voltage":dbl, "Current":dbl, "Current Rate":dbl, "Field":dbl, "Field Rate":dbl, "Persistant Current":dbl, "Persistant Field":dbl, "Target Current":dbl, "Target Field":dbl, "Target Current Rate":dbl, "Target Field Rate":dbl, "Switch Heater Status (SWHT)":string, "Switch Heater Status (SWHN)":string}
  T33 = typedef "Mercury iXX.lvlib/Magnet.lvlib/Identifier.ctl" = string
  T34 = cluster{"time":timestamp, "code":i32, "source":string}[]
  T35 = typedef "LVRectTypeDef.ctl" = cluster{"Left":i16, "Top":i16, "Right":i16, "Bottom":i16}
  T36 = cluster{"Hold":bool, "Clamp":bool, "To Set":bool, "To Zero":bool, "Send to IPS":bool, "PS Heat":bool, "Lambda":bool}
  T37 = typedef "Mercury iXX.lvlib/Magnet.lvlib/PSU Actions.ctl" = string
  T38 = typedef "Mercury iXX.lvlib/Magnet.lvlib/Switch Heater.ctl" = string
  T39 = typedef "Mercury iXX.lvlib/ISOBus Address.ctl" = i32
  T40 = typedef "Mercury iXX.lvlib/Response String.ctl" = string
  T41 = enum32{"invalid app kind", "Development System", "Run Time System", "Student Edition", "Embedded LabVIEW", "Evaluation", "Custom"}
  T42 = cluster{"time":timestamp, "code":i32, "source":string}
  T43 = enum32{"Invalid", "Standard", "Closed", "Hidden", "Minimized", "Maximized"}
  T44 = cluster{"Magnet Field":dbl, "PS Field":dbl, "Target Field":dbl, "Target Field Rate":dbl, "Voltage":dbl, "Current":dbl}
  T45 = typedef "Mercury iXX.lvlib/Comms Transport Layer.ctl" = enum16{"Ethernet TCP/IP", "USB", "ISOBus - RS-232", "GPIB"}
  T46 = typedef "Mercury iXX.lvlib/Query Dynamic Reference.ctl" = refnum<vi>
  T47 = typedef "Mercury iXX.lvlib/Mercury Reference.ctl" = cluster{"Comms":refnum<visa-resource-name>, "Device ID":string[], "Comms Layer":T45, "Command":string, "Query reference":T46}
  T48 = cluster{"Core":cluster{"Current VI Reference":refnum<vi>, "Close Panel on Exit?":bool}, "Mercury ITC Ref":cluster{"Comms":refnum<visa-resource-name>, "Device ID":string[], "Comms Layer":T45, "Command":string, "Query reference":T46}, "Mercury IPS Ref":T47, "sentinel":bool, "Error Log":cluster{"time":timestamp, "code":i32, "source":string}[]}
  T49 = typedef "Mercury-1820-API.lvlib/Actions.ctl" = cluster{"Hold":bool, "Clamp":bool, "To Set":bool, "To Zero":bool, "Send to IPS":bool, "PS Heat":bool, "Lambda":bool}
  T50 = typedef "Mercury-1820-API.lvlib/Targets.ctl" = cluster{"Target Field (T)":dbl, "Target Field Rate (T/min)":dbl}
  T51 = cluster{"Target Field (T)":dbl, "Target Field Rate (T/min)":dbl}
  T52 = cluster{"Comms":refnum<visa-resource-name>, "Device ID":string[], "Comms Layer":T45, "Command":string, "Query reference":T46}
  T53 = typedef "Filtered Error Details - Cluster__ogtk.ctl" = cluster{"code":i32, "source":string}
  T54 = cluster{"Current VI Reference":refnum<vi>, "Close Panel on Exit?":bool}
  T55 = typedef "Mercury iXX.lvlib/System.lvlib/User Mode.ctl" = string
  T56 = typedef "Mercury iXX.lvlib/Magnet.lvlib/Output Configuration.ctl" = string
  T57 = typedef "Mercury-1820-API.lvlib/Status.ctl" = cluster{"Magnet Field":dbl, "PS Field":dbl, "Target Field":dbl, "Target Field Rate":dbl, "Voltage":dbl, "Current":dbl, "Switch":bool, "Mercury State":string}
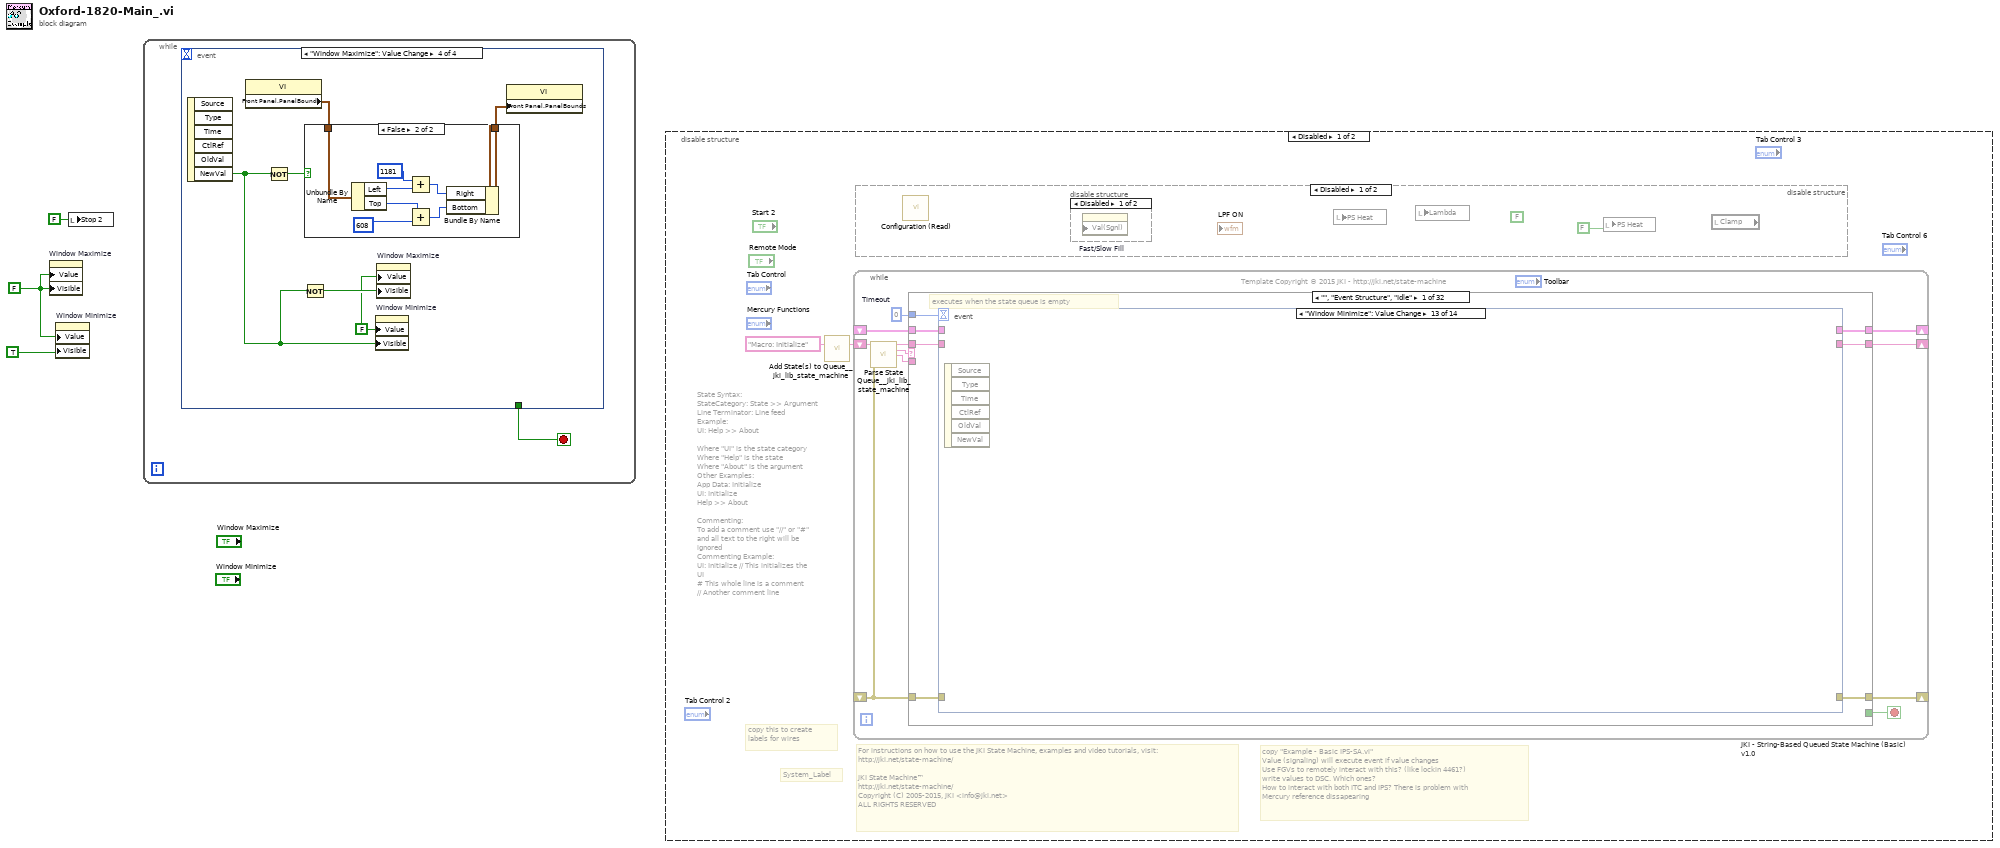
[diagram p0: block diagram]
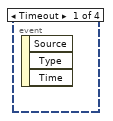
[diagram p2: hidden frame]
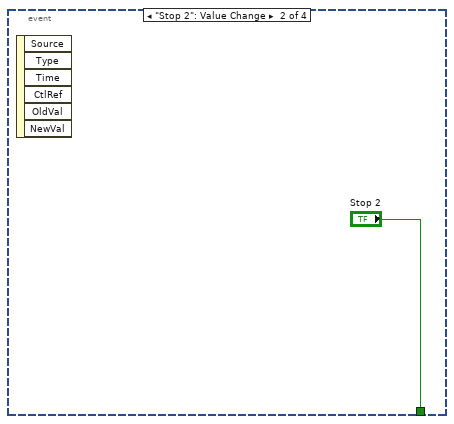
[diagram p3: hidden frame]
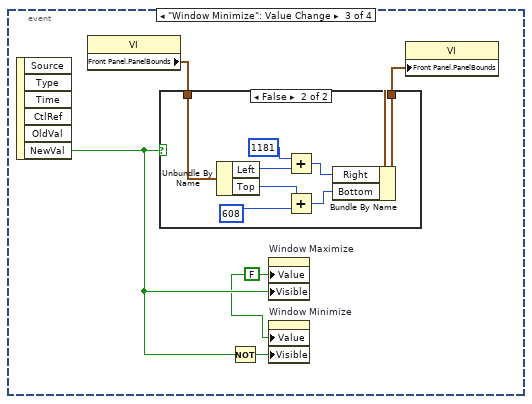
[diagram p4: hidden frame]
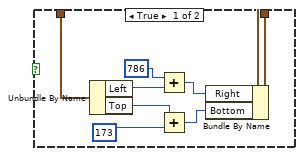
[diagram p5: hidden frame]
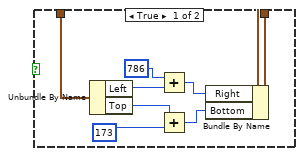
[diagram p6: hidden frame]
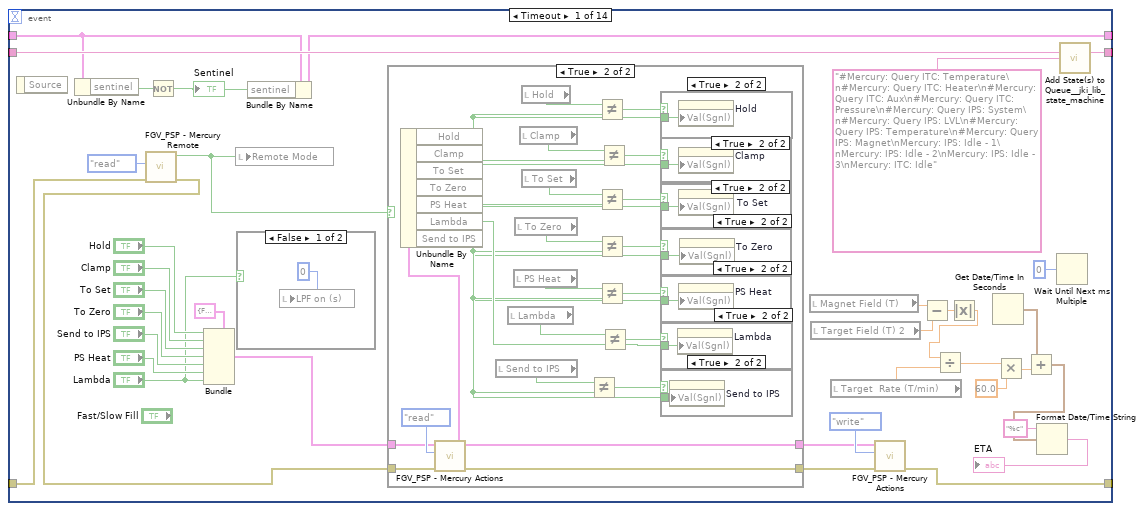
[diagram p9: hidden frame]
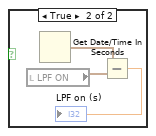
[diagram p10: hidden frame]
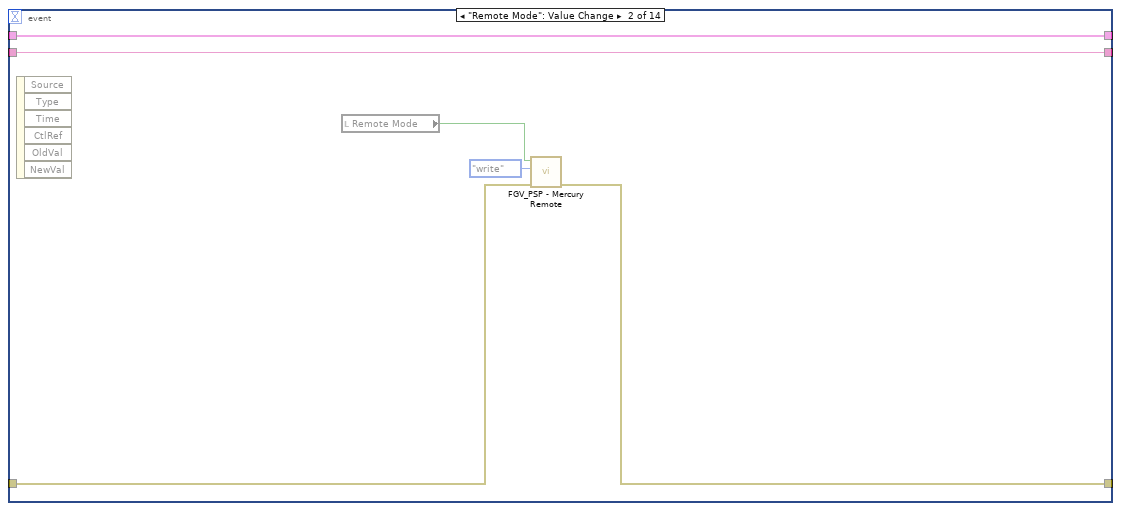
[diagram p19: hidden frame]
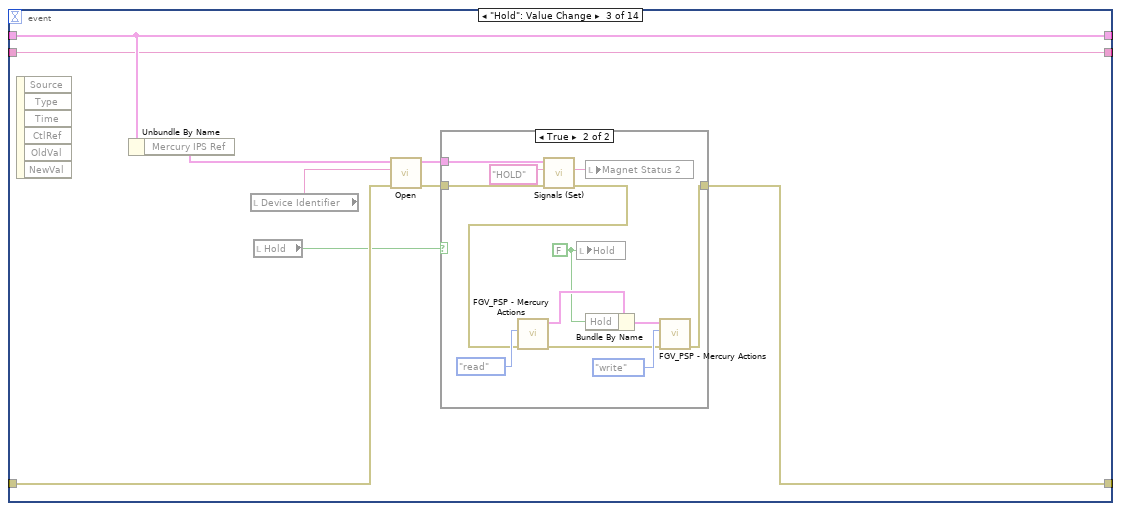
[diagram p20: hidden frame]
diagram:
  w1 = FALSE ("Visible")
  n1 = property on="Window Maximize" class="Bool (strict)"("Value"=w1, "Visible"=w1) -> ()  [unwired: 2 in, 2 out]
  n2 = property on="Window Minimize" class="Bool (strict)"("Value"=w1, "Visible"=TRUE) -> ()  [unwired: 2 in, 2 out]
  n3 = local write "Stop 2"(FALSE ("Stop 2")) -> ()
  n4 = while {
    stop <- w4 stop-if-true
    n5 = event shown="[3] \"Window Maximize\": Value Change" {
      selector: _ -> [_ _ _ _]
      dyn-events: _ -> [_ _ _ _]
      timeout: _ -> [_ _ _ _]
      tunnel: [_ "Stop 2" _ _] -> w4
      event Timeout {
        n6 = event-data() -> ()  [unwired: 1 in, 3 out]
      }
      event "Stop 2": Value Change {
        n7 = event-data() -> ()  [unwired: 1 in, 6 out]
      }
      event "Window Minimize": Value Change {
        w6 = FALSE ("Window Maximize")
        n8 = event-data() -> ("NewVal"=w7:bool)  [unwired: 1 in, 5 out]
        n9 = property class="VI"() -> ("Front Panel.PanelBounds"=w10:T35)  [unwired: 2 in, 2 out]
        n10 = case shown="False" w7 {
          tunnel: w10 -> [w18 w26]
          tunnel: [w17 w25] -> w9
          frame True {
            n11 = Unbundle By Name(w18) -> ("Left"=w16:i16, "Top"=w14:i16)
            n12 = Add(x=i16 786 ("x 6"), y=w16) -> (x+y=w15:i16)
            n13 = Add(x=w14, y=i16 173 ("x 5")) -> (x+y=w13:i16)
            n14 = Bundle By Name(cluster=w18, "Right"=w15, "Bottom"=w13) -> (w17:T35)
          }
          frame False {
            n15 = Unbundle By Name(w26) -> ("Left"=w24:i16, "Top"=w22:i16)
            n16 = Add(x=i16 1181 ("x 8"), y=w24) -> (x+y=w23:i16)
            n17 = Add(x=w22, y=i16 608 ("x 7")) -> (x+y=w21:i16)
            n18 = Bundle By Name(cluster=w26, "Right"=w23, "Bottom"=w21) -> (w25:T35)
          }
        }
        n19 = Not(x=w7) -> (.not. x?=w8:bool)
        n20 = property on="Window Maximize" class="Bool (strict)"("Value"=w6, "Visible"=w7) -> ()  [unwired: 2 in, 2 out]
        n21 = property on="Window Minimize" class="Bool (strict)"("Value"=w6, "Visible"=w8) -> ()  [unwired: 2 in, 2 out]
        n22 = property class="VI"("Front Panel.PanelBounds"=w9) -> ()  [unwired: 2 in, 2 out]
      }
      event "Window Maximize": Value Change {
        w27 = FALSE ("Window Minimize")
        n23 = event-data() -> ("NewVal"=w28:bool)  [unwired: 1 in, 5 out]
        n24 = property class="VI"() -> ("Front Panel.PanelBounds"=w32:T35)  [unwired: 2 in, 2 out]
        n25 = Not(x=w28) -> (.not. x?=w30:bool)
        n26 = Not(x=w28) -> (.not. x?=w29:bool)
        n27 = case shown="False" w30 {
          tunnel: w32 -> [w40 w48]
          tunnel: [w39 w47] -> w31
          frame True {
            n28 = Unbundle By Name(w40) -> ("Left"=w38:i16, "Top"=w36:i16)
            n29 = Add(x=i16 786 ("x 6"), y=w38) -> (x+y=w37:i16)
            n30 = Add(x=w36, y=i16 173 ("x 5")) -> (x+y=w35:i16)
            n31 = Bundle By Name(cluster=w40, "Right"=w37, "Bottom"=w35) -> (w39:T35)
          }
          frame False {
            n32 = Unbundle By Name(w48) -> ("Left"=w46:i16, "Top"=w44:i16)
            n33 = Add(x=i16 1181 ("x 8"), y=w46) -> (x+y=w45:i16)
            n34 = Add(x=w44, y=i16 608 ("x 7")) -> (x+y=w43:i16)
            n35 = Bundle By Name(cluster=w48, "Right"=w45, "Bottom"=w43) -> (w47:T35)
          }
        }
        n36 = property on="Window Minimize" class="Bool (strict)"("Value"=w27, "Visible"=w28) -> ()  [unwired: 2 in, 2 out]
        n37 = property on="Window Maximize" class="Bool (strict)"("Value"=w27, "Visible"=w29) -> ()  [unwired: 2 in, 2 out]
        n38 = property class="VI"("Front Panel.PanelBounds"=w31) -> ()  [unwired: 2 in, 2 out]
      }
    }
  }
  n39 = disable-structure shown="Disabled" {
    frame Disabled {
      # "copy \"Example - Basic IPS-SA.vi\"\nValue (signaling) will execute event if value changes\nUse FGVs to remotely interact with this? (like lockin 4461?)\nwrite values to DSC. Which ones?\nHow to interact with both ITC and IPS? There is problem with \nMercury reference dissapearing"
      # "For instructions on how to use the JKI State Machine, examples and video tutorials, visit:\nhttp://jki.net/state-machine/\n\nJKI State Machine™\nhttp://jki.net/state-machine/\nCopyright (C) 2005-2015, JKI <info@jki.net>\nALL RIGHTS RESERVED"
      # "State Syntax:\nStateCategory: State >> Argument\nLine Terminator: Line feed\nExample:\nUI: Help >> About\n\nWhere \"UI\" is the state category\nWhere \"Help\" is the state\nWhere \"About\" is the argument\nOther Examples:\nApp Data: Initialize\nUI: Initialize\nHelp >> About\n\nCommenting:\nTo add a comment use \"//\" or \"#\" and all text to the right will be ignored\nCommenting Example:\nUI: Initialize // This initializes the UI\n# This whole line is a comment\n// Another comment line"
      # "copy this to create labels for wires"
      # "System_Label"
      n40 = call <vilib>:"Add State(s) to Queue__jki_lib_state_machine.vi"("State(s) in (\"\")"="Macro: Initialize") -> ("States Out"=w50:string)  [unwired: 14 in]
      n41 = while "JKI - String-Based Queued State Machine (Basic) v1.0" {
        shift-right: [w55] -> _
        shift-left: _ -> [w54]
        shift-right: [w58] -> _
        shift-left: _ -> [w52]
        shift-right: [w57] -> _
        shift-left: w50 -> [w59]
        stop <- w56 stop-if-true
        w53 = 0  # Timeout
        # "Template Copyright © 2015 JKI - http://jki.net/state-machine"
        n42 = call <vilib>:"Parse State Queue__jki_lib_state_machine.vi"("State Queue"=w59, "Error In (no error)"=w52) -> ("Remaining States"=w61:string, "Current State"=w62:string, "Arguments"=w60:string)  [unwired: 11 in]
        n43 = case shown="\"\", \"Event Structure\", \"Idle\"" w62 {
          selector: w62 -> [_ _ w399 _ _ _ _ _ _ _ _ _ _ _ _ _ _ _ _ _ _ _ _ _ _ _ _ _ _ _ _ _]
          tunnel: w61 -> [w69 w398 w403 w421 w438 w443 w447 w456 w462 w466 w478 w485 w496 w522 w527 w542 w546 w569 w613 w659 w701 w748 w769 w814 w855 w902 w943 w986 w1046 w1088 w1092 w1097]
          tunnel: w60 -> [_ _ _ _ _ _ _ _ _ _ _ w480 w490 _ _ _ _ _ _ _ _ _ _ _ _ _ _ _ _ _ _ _]
          tunnel: w54 -> [w65 w395 w401 w412 w424 w441 w444 _ w457 w463 w476 w483 w492 w519 w525 w540 w543 w564 w611 w658 w665 w708 w755 w812 w854 w901 w942 w985 w1045 w1087 w1091 w1096]
          tunnel: [w63 w396 w405 w418 errorcluster {"status"=FALSE, "code"=0, "source"=""} ("error out") w440 w445 w449 w458 w464 w472 w481 w493 w520 w524 w528 w544 w548 w573 w620 w662 w711 w756 w776 w821 w860 w909 w948 w1024 w1062 w1090 w1094] -> w58
          tunnel: [w68 w397 w402 w420 w437 w442 w446 w455 w461 w465 w477 w484 w495 w521 w526 w541 w545 w568 w612 w660 w702 w749 w770 w813 w856 w903 w944 w987 w1047 w1089 w1093 w1098] -> w57
          tunnel: [_ _ _ _ _ TRUE _ _ _ _ _ _ _ _ _ _ _ _ _ _ _ _ _ _ _ _ _ _ _ _ _ _] -> w56
          tunnel: [w67 w395 w401 w419 w423 w441 w444 w454 w457 w463 w476 w483 w492 w519 w525 w540 w543 w563 w611 w658 w665 w708 w755 w812 w854 w901 w942 w985 w1045 w1087 w1091 w1096] -> w55
          tunnel: w53 -> [w66 _ _ _ _ _ _ _ _ _ _ _ _ _ _ _ _ _ _ _ _ _ _ _ _ _ _ _ _ _ _ _]
          tunnel: w52 -> [w64 w396 w404 w418 w433 w440 w445 w449 w459 w464 w468 w482 w494 w520 w524 w530 w544 w556 w575 w621 w668 w710 w750 w778 w823 w857 w904 w984 w1025 w1063 w1090 w1095]
          frame "", "Event Structure", "Idle" {
            # "executes when the state queue is empty"
            n44 = event shown="[12] \"Window Minimize\": Value Change" {
              selector: _ -> [_ _ _ _ _ _ _ _ _ _ _ _ _ _]
              dyn-events: _ -> [_ _ _ _ _ _ _ _ _ _ _ _ _ _]
              timeout: w66 -> [_ _ _ _ _ _ _ _ _ _ _ _ _ _]
              tunnel: w69 -> [w106 w148 w159 w182 w203 w226 w251 w294 w333 w352 w363 w388 _ w394]
              tunnel: [w105 w148 w159 w182 w203 w226 w251 w294 w333 w352 w363 w387 _ w393] -> w68
              tunnel: [w100 w147 w160 w183 w204 w225 w252 w290 w332 w346 w365 w385 _ w391] -> w67
              tunnel: w65 -> [w101 w147 w160 w183 w204 w225 w252 w290 w332 w346 w365 w385 _ w391]
              tunnel: w64 -> [w84 w150 w156 w178 w198 w220 w246 w293 w330 w350 w364 w386 _ w392]
              tunnel: [w94 w149 w158 w176 w205 w227 w250 w291 w324 w337 w356 w386 _ w392] -> w63
              event Timeout {
                n45 = event-data() -> ()  [unwired: 1 in, 1 out]
                n46 = Unbundle By Name(w101) -> ("sentinel"=w103:bool)
                n47 = call <userlib>:"FGV_PSP - Mercury Remote.vi"("error in"=w84, "Function"=enum16{"write", "read"}."read") -> ("error out"=w83:errorcluster, "Remote"=w82:bool)  [unwired: 4 in]
                n48 = Not(x=w103) -> (.not. x?=w102:bool)
                "Sentinel" <- w102
                n49 = Bundle(cluster=T36 {"Hold"=FALSE, "Clamp"=FALSE, "To Set"=FALSE, "To Zero"=FALSE, "Send to IPS"=FALSE, "PS Heat"=FALSE, "Lambda"=FALSE}, "Hold"="Hold", "Clamp"="Clamp", "To Set"="To Set", "To Zero"="To Zero", "Send to IPS"="Send to IPS", "PS Heat"="PS Heat", "Lambda"="Lambda") -> (w92:T36)
                n50 = local write "Remote Mode"(w82) -> ()
                n51 = case shown="False" "Lambda" {
                  frame False {
                    n52 = local write "LPF on (s)"(0 ("LPF on (s)")) -> ()
                  }
                  frame True {
                    n53 = local read "LPF ON"() -> (w110:timestamp)
                    n54 = Get Date/Time In Seconds() -> (seconds since 1Jan1904=w109:timestamp)
                    n55 = Subtract(x=w109, y=w110) -> (x-y=→"LPF on (s)":dbl)
                  }
                }
                n56 = Bundle By Name(cluster=w101, "sentinel"=w102) -> (w100:T48)
                n57 = case shown="True" w82 {
                  tunnel: [w111 w137] -> w93
                  tunnel: w83 -> [w111 w136]
                  tunnel: w92 -> [w112 w135]
                  tunnel: [w112 w127] -> w91
                  frame False {
                  }
                  frame True {
                    n58 = call <userlib>:"FGV_PSP - Mercury Actions.vi"("error in"=w136, "Function"=enum16{"write", "read"}."read", "Actions"=w135) -> ("error out"=w137:errorcluster, "Actions"=w127:T49)  [unwired: 3 in]
                    n59 = Unbundle By Name(w127) -> ("Hold"=w119:bool, "Clamp"=w121:bool, "To Set"=w122:bool, "To Zero"=w123:bool, "PS Heat"=w124:bool, "Lambda"=w125:bool, "Send to IPS"=w126:bool)
                    n60 = local read "Send to IPS"() -> (w120:bool)
                    n61 = local read "Lambda"() -> (w118:bool)
                    n62 = local read "PS Heat"() -> (w117:bool)
                    n63 = local read "To Zero"() -> (w116:bool)
                    n64 = local read "Clamp"() -> (w114:bool)
                    n65 = local read "Hold"() -> (w113:bool)
                    n66 = local read "To Set"() -> (w115:bool)
                    n67 = Not Equal?(x=w120, y=w126) -> (x != y?=w128:bool)
                    n68 = Not Equal?(x=w113, y=w119) -> (x != y?=w134:bool)
                    n69 = Not Equal?(x=w115, y=w122) -> (x != y?=w132:bool)
                    n70 = Not Equal?(x=w116, y=w123) -> (x != y?=w131:bool)
                    n71 = Not Equal?(x=w117, y=w124) -> (x != y?=w130:bool)
                    n72 = Not Equal?(x=w114, y=w121) -> (x != y?=w133:bool)
                    n73 = Not Equal?(x=w118, y=w125) -> (x != y?=w129:bool)
                    n74 = case shown="True" w134 {
                      tunnel: w119 -> [_ w145]
                      frame False {
                      }
                      frame True {
                        n75 = property on="Hold" class="Bool (strict)"("Val(Sgnl)"=w145) -> ()  [unwired: 2 in, 2 out]
                      }
                    }
                    n76 = case shown="True" w133 {
                      tunnel: w121 -> [_ w144]
                      frame False {
                      }
                      frame True {
                        n77 = property on="Clamp" class="Bool (strict)"("Val(Sgnl)"=w144) -> ()  [unwired: 2 in, 2 out]
                      }
                    }
                    n78 = case shown="True" w132 {
                      tunnel: w122 -> [_ w143]
                      frame False {
                      }
                      frame True {
                        n79 = property on="To Set" class="Bool (strict)"("Val(Sgnl)"=w143) -> ()  [unwired: 2 in, 2 out]
                      }
                    }
                    n80 = case shown="True" w131 {
                      tunnel: w123 -> [_ w142]
                      frame False {
                      }
                      frame True {
                        n81 = property on="To Zero" class="Bool (strict)"("Val(Sgnl)"=w142) -> ()  [unwired: 2 in, 2 out]
                      }
                    }
                    n82 = case shown="True" w130 {
                      tunnel: w124 -> [_ w141]
                      frame False {
                      }
                      frame True {
                        n83 = property on="PS Heat" class="Bool (strict)"("Val(Sgnl)"=w141) -> ()  [unwired: 2 in, 2 out]
                      }
                    }
                    n84 = case shown="True" w129 {
                      tunnel: w125 -> [_ w140]
                      frame False {
                      }
                      frame True {
                        n85 = property on="Lambda" class="Bool (strict)"("Val(Sgnl)"=w140) -> ()  [unwired: 2 in, 2 out]
                      }
                    }
                    n86 = case shown="True" w128 {
                      tunnel: w126 -> [_ w139]
                      frame False {
                      }
                      frame True {
                        n87 = property on="Send to IPS" class="Bool (strict)"("Val(Sgnl)"=w139) -> ()  [unwired: 2 in, 2 out]
                      }
                    }
                  }
                }
                n88 = local read "Magnet Field (T)"() -> (w80:dbl)
                n89 = local read "Target Field (T) 2"() -> (w79:dbl)
                n90 = local read "Target  Rate (T/min)"() -> (w81:dbl)
                n91 = call <userlib>:"FGV_PSP - Mercury Actions.vi"("error in"=w93, "Function"=enum16{"write", "read"}."write", "Actions"=w91) -> ("error out"=w94:errorcluster)  [unwired: 3 in, 1 out]
                n92 = Subtract(x=w80, y=w79) -> (x-y=w78:dbl)
                n93 = Absolute Value(x=w78) -> (abs(x)=w77:dbl)
                n94 = Divide(x=w77, y=w81) -> (x/y=w76:dbl)
                n95 = Get Date/Time In Seconds() -> (seconds since 1Jan1904=w73:timestamp)
                n96 = Multiply(x=w76, y=60.0) -> (x*y=w74:dbl)
                n97 = Add(x=w73, y=w74) -> (x+y=w72:timestamp)
                n98 = Format Date/Time String(time format string (%c)="%c", seconds (now)=w72) -> (date/time string=→"ETA":string)  [unwired: 1 in]
                n99 = Wait Until Next ms Multiple(millisecond multiple=u32 0) -> ()  [unwired: 1 out]
                n100 = call <vilib>:"Add State(s) to Queue__jki_lib_state_machine.vi"("State(s) in (\"\")"=w106, "State(s) at Back (\"\")"="#Mercury: Query ITC: Temperature\n#Mercury: Query ITC: Heater\n#Mercury: Query ITC: Aux\n#Mercury: Query ITC: Pressure\n#Mercury: Query IPS: System\n#Mercury: Query IPS: LVL\n#Mercury: Query IPS: Temperature\n#Mercury: Query IPS: Magnet\nMercury: IPS: Idle - 1\nMercury: IPS: Idle - 2\nMercury: IPS: Idle - 3\nMercury: ITC: Idle" ("State(s) at Back (\"\")")) -> ("States Out"=w105:string)  [unwired: 13 in]
              }
              event "Remote Mode": Value Change {
                n101 = event-data() -> ()  [unwired: 1 in, 6 out]
                n102 = local read "Remote Mode"() -> (w146:bool)
                n103 = call <userlib>:"FGV_PSP - Mercury Remote.vi"("error in"=w150, "Function"=enum16{"write", "read"}."write", "Remote"=w146) -> ("error out"=w149:errorcluster)  [unwired: 3 in, 1 out]
              }
              event "Hold": Value Change {
                n104 = event-data() -> ()  [unwired: 1 in, 6 out]
                n105 = Unbundle By Name(w160) -> ("Mercury IPS Ref"=w154:T47)
                n106 = local read "Device Identifier"() -> (w155:T33)
                n107 = local read "Hold"() -> (w152:bool)
                n108 = call-poly <instrlib>:"Open.vi"("error in (no error)"=w156, "Device Identifier"=w155, "Mercury Reference In"=w154) -> ("error out"=w157:errorcluster, "Mercury Reference Out"=w153:T47)  [unwired: 7 out]
                n109 = case shown="True" w152 {
                  tunnel: [w161 w163] -> w158
                  tunnel: w157 -> [w161 w172]
                  tunnel: w153 -> [_ w171]
                  frame False {
                  }
                  frame True {
                    w168 = FALSE ("Hold")
                    n110 = call-poly <instrlib>:"Signals (Set).vi"("error in"=w172, "PSU Act Stat"=T37 "HOLD", "Mercury Reference In"=w171) -> ("error out"=w162:errorcluster, "Response"=w170:T40)  [unwired: 1 in, 6 out]
                    n111 = call <userlib>:"FGV_PSP - Mercury Actions.vi"("error in"=w162, "Function"=enum16{"write", "read"}."read") -> ("error out"=w165:errorcluster, "Actions"=w169:T49)  [unwired: 4 in]
                    n112 = local write "Hold"(w168) -> ()
                    n113 = local write "Magnet Status 2"(w170) -> ()
                    n114 = Bundle By Name(cluster=w169, "Hold"=w168) -> (w167:T49)
                    n115 = call <userlib>:"FGV_PSP - Mercury Actions.vi"("error in"=w165, "Function"=enum16{"write", "read"}."write", "Actions"=w167) -> ("error out"=w163:errorcluster)  [unwired: 3 in, 1 out]
                  }
                }
              }
              event "Clamp": Value Change {
                n116 = event-data() -> ()  [unwired: 1 in, 6 out]
                n117 = Unbundle By Name(w183) -> ("Mercury IPS Ref"=w177:T47)
                n118 = local read "Device Identifier"() -> (w181:T33)
                n119 = Two Button Dialog(message="You have pushed the clamp button\nAre you sure?") -> (T button?=w174:bool)  [unwired: 2 in]
                n120 = call-poly <instrlib>:"Open.vi"("error in (no error)"=w178, "Device Identifier"=w181, "Mercury Reference In"=w177) -> ("error out"=w180:errorcluster, "Mercury Reference Out"=w179:T47)  [unwired: 7 out]
                n121 = case shown="True" w174 {
                  tunnel: w180 -> [w184 w194]
                  tunnel: w179 -> [_ w193]
                  tunnel: [w184 w186] -> w176
                  frame False {
                  }
                  frame True {
                    w185 = FALSE
                    n122 = call-poly <instrlib>:"Signals (Set).vi"("error in"=w194, "PSU Act Stat"=T37 "CLMP", "Mercury Reference In"=w193) -> ("error out"=w187:errorcluster, "Response"=w195:T40)  [unwired: 1 in, 6 out]
                    n123 = call <userlib>:"FGV_PSP - Mercury Actions.vi"("error in"=w187, "Function"=enum16{"write", "read"}."read") -> ("error out"=w189:errorcluster, "Actions"=w192:T49)  [unwired: 4 in]
                    n124 = local write "Clamp"(w185) -> ()
                    n125 = Bundle By Name(cluster=w192, "Clamp"=w185) -> (w191:T49)
                    n126 = local write "Magnet Status 2"(w195) -> ()
                    n127 = call <userlib>:"FGV_PSP - Mercury Actions.vi"("error in"=w189, "Function"=enum16{"write", "read"}."write", "Actions"=w191) -> ("error out"=w186:errorcluster)  [unwired: 3 in, 1 out]
                  }
                }
              }
              event "To Set": Value Change {
                n128 = event-data() -> ()  [unwired: 1 in, 6 out]
                n129 = Unbundle By Name(w204) -> ("Mercury IPS Ref"=w200:T47)
                n130 = local read "Device Identifier"() -> (w199:T33)
                n131 = call-poly <instrlib>:"Open.vi"("error in (no error)"=w198, "Device Identifier"=w199, "Mercury Reference In"=w200) -> ("error out"=w201:errorcluster, "Mercury Reference Out"=w202:T47)  [unwired: 7 out]
                n132 = local read "To Set"() -> (w197:bool)
                n133 = case shown="True" w197 {
                  tunnel: [w206 w208] -> w205
                  tunnel: w202 -> [_ w216]
                  tunnel: w201 -> [w206 w215]
                  frame False {
                  }
                  frame True {
                    w207 = FALSE
                    n134 = call-poly <instrlib>:"Signals (Set).vi"("error in"=w215, "PSU Act Stat"=T37 "RTOS", "Mercury Reference In"=w216) -> ("error out"=w209:errorcluster, "Response"=w217:T40)  [unwired: 1 in, 6 out]
                    n135 = call <userlib>:"FGV_PSP - Mercury Actions.vi"("error in"=w209, "Function"=enum16{"write", "read"}."read") -> ("error out"=w211:errorcluster, "Actions"=w214:T49)  [unwired: 4 in]
                    n136 = Bundle By Name(cluster=w214, "To Set"=w207) -> (w213:T49)
                    n137 = local write "To Set"(w207) -> ()
                    n138 = local write "Magnet Status 2"(w217) -> ()
                    n139 = call <userlib>:"FGV_PSP - Mercury Actions.vi"("error in"=w211, "Function"=enum16{"write", "read"}."write", "Actions"=w213) -> ("error out"=w208:errorcluster)  [unwired: 3 in, 1 out]
                  }
                }
              }
              event "To Zero": Value Change {
                n140 = event-data() -> ()  [unwired: 1 in, 6 out]
                n141 = Unbundle By Name(w225) -> ("Mercury IPS Ref"=w222:T47)
                n142 = local read "Device Identifier"() -> (w221:T33)
                n143 = local read "To Zero"() -> (w219:bool)
                n144 = call-poly <instrlib>:"Open.vi"("error in (no error)"=w220, "Device Identifier"=w221, "Mercury Reference In"=w222) -> ("error out"=w223:errorcluster, "Mercury Reference Out"=w224:T47)  [unwired: 7 out]
                n145 = case shown="True" w219 {
                  tunnel: [w228 w231] -> w227
                  tunnel: w224 -> [_ w238]
                  tunnel: w223 -> [w228 w237]
                  frame False {
                  }
                  frame True {
                    w229 = FALSE
                    n146 = call-poly <instrlib>:"Signals (Set).vi"("error in"=w237, "PSU Act Stat"=T37 "RTOZ", "Mercury Reference In"=w238) -> ("error out"=w232:errorcluster, "Response"=w239:T40)  [unwired: 1 in, 6 out]
                    n147 = call <userlib>:"FGV_PSP - Mercury Actions.vi"("error in"=w232, "Function"=enum16{"write", "read"}."read") -> ("error out"=w234:errorcluster, "Actions"=w230:T49)  [unwired: 4 in]
                    n148 = Bundle By Name(cluster=w230, "To Zero"=w229) -> (w236:T49)
                    n149 = local write "To Zero"(w229) -> ()
                    n150 = local write "Magnet Status 2"(w239) -> ()
                    n151 = call <userlib>:"FGV_PSP - Mercury Actions.vi"("error in"=w234, "Function"=enum16{"write", "read"}."write", "Actions"=w236) -> ("error out"=w231:errorcluster)  [unwired: 3 in, 1 out]
                  }
                }
              }
              event "PS Heat": Value Change {
                n152 = event-data() -> ("NewVal"=w241:bool)  [unwired: 1 in, 5 out]
                n153 = local read "Device Identifier"() -> (w247:T33)
                n154 = Unbundle By Name(w252) -> ("Mercury IPS Ref"=w248:T47)
                n155 = call-poly <instrlib>:"Open.vi"("error in (no error)"=w246, "Device Identifier"=w247, "Mercury Reference In"=w248) -> ("error out"=w243:errorcluster, "Mercury Reference Out"=w244:T47)  [unwired: 7 out]
                n156 = call-poly <instrlib>:"Signals (Read).vi"("error in"=w243, "Mercury Reference In"=w244) -> ("error out"=w254:errorcluster, "Current"=w249:dbl, "Mercury Reference Out"=w253:T47)  [unwired: 1 in, 6 out]
                n157 = call-poly <instrlib>:"Signals (Read).vi"("error in"=w254, "Mercury Reference In"=w253) -> ("error out"=w255:errorcluster, "Persistant Current"=w245:dbl, "Mercury Reference Out"=w256:T47)  [unwired: 1 in, 6 out]
                n158 = Subtract(x=w245, y=w249) -> (x-y=w257:dbl)
                n159 = Absolute Value(x=w257) -> (abs(x)=w258:dbl)
                n160 = Less?(x=w258, y=0.1) -> (x < y?=w260:bool)
                n161 = case shown="False" w260 {
                  selector: w260 -> [_ w263]
                  tunnel: [w262 w263] -> w242
                  frame False {
                    n162 = Two Button Dialog(message="The magnet current is more\nthan 0.1A different to the\nPSU output current.  It is not\nadvisable to switch on the\nswitch heater unless these\ncurrents are equal!") -> (T button?=w262:bool)  [unwired: 2 out]
                  }
                  frame True {
                  }
                }
                n163 = case shown="True" w242 {
                  tunnel: w256 -> [_ w283]
                  tunnel: w255 -> [w264 w282]
                  tunnel: [w264 w276] -> w250
                  tunnel: w241 -> [_ w266]
                  frame False {
                  }
                  frame True {
                    n164 = call-poly <instrlib>:"Signals (Read).vi"("error in"=w282, "Mercury Reference In"=w283) -> ("error out"=w271:errorcluster, "Mercury Reference Out"=w267:T47)  [unwired: 1 in, 7 out]
                    n165 = call <userlib>:"Wait (ms)__ogtk.vi"("error in (no error)"=w271, "milliseconds to wait"=u32 100 ("millisecond multiple")) -> ("error out"=w270:errorcluster)  [unwired: 8 in, 1 out]
                    n166 = Select(t=T38 "" ("Set Switch Heater"), s=w266, f=T38 "" ("Set Switch Heater")) -> (s? t:f=w268:T38)
                    n167 = call-poly <instrlib>:"Signals (Set).vi"("error in"=w270, "Switch Heater Status"=w268, "Mercury Reference In"=w267) -> ("error out"=w284:errorcluster, "Response"=w273:T40, "Mercury Reference Out"=w285:T47)  [unwired: 1 in, 5 out]
                    n168 = local write "Magnet Status 2"(w273) -> ()
                    n169 = call-poly <instrlib>:"Configuration (Read).vi"("error in"=w284, "Mercury Reference In"=w285) -> ("error out"=w265:errorcluster, "Time"=→"Switch Time":string)  [unwired: 1 in, 7 out]
                    n170 = call <userlib>:"FGV_PSP - Mercury Actions.vi"("error in"=w265, "Function"=enum16{"write", "read"}."read") -> ("error out"=w279:errorcluster, "Actions"=w277:T49)  [unwired: 4 in]
                    n171 = Bundle By Name(cluster=w277, "PS Heat"=w266) -> (w281:T49)
                    n172 = call <userlib>:"FGV_PSP - Mercury Actions.vi"("error in"=w279, "Function"=enum16{"write", "read"}."write", "Actions"=w281) -> ("error out"=w276:errorcluster)  [unwired: 3 in, 1 out]
                  }
                }
              }
              event "Send to IPS": Value Change {
                n173 = event-data() -> ()  [unwired: 1 in, 6 out]
                n174 = local read "Device Identifier"() -> (w289:T33)
                n175 = Unbundle By Name(w290) -> ("Mercury IPS Ref"=w288:T47)
                n176 = local read "Send to IPS"() -> (w286:bool)
                n177 = call-poly <instrlib>:"Open.vi"("error in (no error)"=w293, "Device Identifier"=w289, "Mercury Reference In"=w288) -> ("error out"=w292:errorcluster, "Mercury Reference Out"=w287:T47)  [unwired: 7 out]
                n178 = case shown="True" w286 {
                  tunnel: w292 -> [w295 w314]
                  tunnel: [w295 w298] -> w291
                  tunnel: w287 -> [_ w312]
                  frame False {
                  }
                  frame True {
                    w297 = FALSE
                    n179 = local read "Remote Mode"() -> (w310:bool)
                    n180 = case shown="True" w310 {
                      tunnel: "Target Field (T) 2" -> [w316 _]
                      tunnel: "Target Rate (T/min)" -> [w315 _]
                      tunnel: [w316 w318] -> w304
                      tunnel: [w315 w317] -> w305
                      frame False {
                      }
                      frame True {
                        n181 = call <userlib>:"FGV_PSP - Mercury Targets.vi"("Function"=enum16{"write", "read"}."read") -> ("Targets"=w319:T50)  [unwired: 5 in, 1 out]
                        n182 = Unbundle(w319) -> ("Target Field (T)"=w318:dbl, "Target Field Rate (T/min)"=w317:dbl)
                      }
                    }
                    n183 = local write "Send to IPS"(w297) -> ()
                    n184 = call-poly <instrlib>:"Signals (Set).vi"("error in"=w314, "Target Field Rate"=w305, "Mercury Reference In"=w312) -> ("error out"=w313:errorcluster, "Mercury Reference Out"=w311:T47)  [unwired: 2 in, 5 out]
                    n185 = local write "Target Field (T) 2"(w304) -> ()
                    n186 = local write "Target Rate (T/min)"(w305) -> ()
                    n187 = Bundle("Target Field (T)"=w304, "Target Field Rate (T/min)"=w305) -> (w307:T51)  [unwired: 1 in]
                    n188 = call-poly <instrlib>:"Signals (Set).vi"("error in"=w313, "Target Field"=w304, "Mercury Reference In"=w311) -> ("error out"=w296:errorcluster)  [unwired: 2 in, 6 out]
                    n189 = call <userlib>:"FGV_PSP - Mercury Actions.vi"("error in"=w296, "Function"=enum16{"write", "read"}."read") -> ("error out"=w301:errorcluster, "Actions"=w299:T49)  [unwired: 4 in]
                    n190 = Bundle By Name(cluster=w299, "Send to IPS"=w297) -> (w303:T49)
                    n191 = call <userlib>:"FGV_PSP - Mercury Actions.vi"("error in"=w301, "Function"=enum16{"write", "read"}."write", "Actions"=w303) -> ("error out"=w298:errorcluster)  [unwired: 3 in, 1 out]
                    n192 = call <userlib>:"FGV_PSP - Mercury Targets.vi"("Function"=enum16{"write", "read"}."write", "Targets"=w307) -> ()  [unwired: 4 in, 2 out]
                  }
                }
              }
              event "Lambda": Value Change {
                # "AUX\nPRES\nHTR\nTEMP"
                n193 = event-data() -> ()  [unwired: 1 in, 6 out]
                n194 = Unbundle By Name(w332) -> ("Mercury ITC Ref"=w331:T52)
                n195 = call-poly <instrlib>:"Open.vi"("error in (no error)"=w330, "Device Identifier"="lambda:LPC", "Mercury Reference In"=w331) -> ("error out"=w327:errorcluster, "Mercury Reference Out"=w326:T47)  [unwired: 7 out]
                n196 = local read "Lambda"() -> (w321:bool)
                n197 = Select(t="ON" ("Sweep Mode"), s=w321, f="OFF" ("Sweep Mode")) -> (s? t:f=w325:string)
                n198 = case shown="False" w321 {
                  frame False {
                    n199 = disable-structure shown="Disabled" {
                      frame Disabled {
                        n200 = property on="Close Needle Valve" class="Bool (strict)"("Val(Sgnl)"=TRUE ("Value (Signaling)")) -> ()  [unwired: 2 in, 2 out]
                      }
                      frame Enabled {
                      }
                    }
                  }
                  frame True {
                  }
                }
                n201 = case shown="False" w321 {
                  frame False {
                    n202 = local write "LPF ON"(timestamp(0 s since 1904-01-01) ("LPF ON")) -> ()
                  }
                  frame True {
                    n203 = Get Date/Time In Seconds() -> (seconds since 1Jan1904=w336:timestamp)
                    n204 = local write "LPF ON"(w336) -> ()
                  }
                }
                n205 = call-poly <instrlib>:"Configuration (Set).vi"("error in"=w327, "Lambda Auto"=w325, "Mercury Reference In"=w326) -> ("error out"=w324:errorcluster, "Response"=w323:T40)  [unwired: 5 in, 2 out]
                n206 = local write "Magnet Status 2"(w323) -> ()
              }
              event "Fast/Slow Fill": Value Change {
                n207 = event-data() -> ()  [unwired: 1 in, 6 out]
                n208 = local read "IPS Devices"() -> (w348:string[])
                n209 = Unbundle By Name(w346) -> ("Mercury IPS Ref"=w351:T47)
                n210 = Index Array(array=w348, index=0) -> (element=w347:string)
                n211 = local read "Fast/Slow Fill"() -> (w344:bool)
                n212 = call-poly <instrlib>:"Open.vi"("error in (no error)"=w350, "Device Identifier"=w347, "Mercury Reference In"=w351) -> ("error out"=w340:errorcluster, "Mercury Reference Out"=w341:T47)  [unwired: 7 out]
                n213 = Select(t="OFF" ("Temperature setpoint"), s=w344, f="ON" ("Temperature setpoint")) -> (s? t:f=w342:string)
                n214 = call-poly <instrlib>:"Configuration (Set).vi"("ISOBUS address"=T39 -1, "error in"=w340, "Delay"=w342, "Mercury Reference In"=w341) -> ("error out"=w337:errorcluster, "Response"=w339:T40)  [unwired: 4 in, 2 out]
                n215 = local write "Magnet Status 2"(w339) -> ()
              }
              event "Close Needle Valve", "Open Needle Valve": Value Change {
                n216 = event-data() -> ()  [unwired: 1 in, 6 out]
                n217 = Unbundle By Name(w365) -> ("Mercury ITC Ref"=w366:T52)
                n218 = Build Array("Close Needle Valve", "Open Needle Valve") -> (w359:bool[])
                n219 = call-poly <instrlib>:"Open.vi"("error in (no error)"=w364, "Device Identifier"="lambda:LPC", "Mercury Reference In"=w366) -> ("error out"=w358:errorcluster, "Mercury Reference Out"=w357:T47)  [unwired: 7 out]
                n220 = Boolean Array To Number(Boolean array=w359) -> (number=w354:u32)
                n221 = case shown="0, Default" w354 {
                  tunnel: w358 -> [w369 w373 w381]
                  tunnel: w357 -> [_ w374 w380]
                  tunnel: [w369 w372 w379] -> w356
                  tunnel: [T40 "" ("Response") w371 w378] -> w355
                  tunnel: [FALSE ("Close Needle Valve") FALSE ("Close Needle Valve") FALSE ("Close Needle Valve")] -> w353
                  frame 0, Default {
                  }
                  frame 1 {
                    n222 = call-poly <instrlib>:"Configuration (Set).vi"("ISOBUS address"=T39 -1, "error in"=w373, "Percentage Open"=0.0, "Mercury Reference In"=w374) -> ("error out"=w372:errorcluster, "Response"=w371:T40)  [unwired: 4 in, 2 out]
                  }
                  frame 2 {
                    n223 = call-poly <instrlib>:"Configuration (Set).vi"("ISOBUS address"=T39 -1, "error in"=w381, "Percentage Open"=100.0, "Mercury Reference In"=w380) -> ("error out"=w379:errorcluster, "Response"=w378:T40)  [unwired: 4 in, 2 out]
                  }
                }
                n224 = local write "Close Needle Valve"(w353) -> ()
                n225 = local write "Open Needle Valve"(w353) -> ()
                n226 = local write "Magnet Status 2"(w355) -> ()
              }
              event "Stop 2": Value Change {
                # "Exit Button Value Change (pressed) Event\n(this executes Macro: Exit to terminate the VI)"
                n227 = event-data() -> ()  [unwired: 1 in, 6 out]
                n228 = call <vilib>:"Add State(s) to Queue__jki_lib_state_machine.vi"("State(s) in Front (\"\")"="Macro: Exit", "State(s) in (\"\")"=w388) -> ("States Out"=w387:string)  [unwired: 13 in]
              }
              event "Window Minimize": Value Change {
                n229 = event-data() -> ()  [unwired: 1 in, 6 out]
              }
              event Panel Close? {
                # "Discard the event because we'll close the front panel ourselves in Macro: Exit"
                # "Close Panel button (pressed) Event\n(this executes Macro: Exit to terminate the VI)"
                n230 = event-data() -> ()  [unwired: 1 in, 1 out]
                n231 = call <vilib>:"Add State(s) to Queue__jki_lib_state_machine.vi"("State(s) in Front (\"\")"="Macro: Exit", "State(s) in (\"\")"=w394) -> ("States Out"=w393:string)  [unwired: 13 in]
                n232 = event-data("Discard?"=TRUE) -> ()  [unwired: 1 in, 1 out]
              }
            }
          }
          frame "---------- Core ----------" {
            # "Do not put any code in this frame.\n(it is a separator no-op)"
            n233 = call <vilib>:"Add State(s) to Queue__jki_lib_state_machine.vi"("State(s) in (\"\")"=w398) -> ("States Out"=w397:string)  [unwired: 14 in]
          }
          frame Default {
            w408 = 42 items=["No error", "Argument error", "Memory is full", "Out of zone", "End of file", "File already open", "Generic file I/O error", "File not found", "File permission error", "Disk is full", "Duplicate path", "Too many files open", "System feature not enabled", "Resource file not found", "Cannot add resource", "Resource not found", "Image not found", "Image memory error", "Pen does not exist", "Config type invalid", "Config token not found", "Config parse error", "Config memory error", "Bad external code format", "Bad external code offset", "External code not present", "Null window", "Destroy window error", "Null menu", "Print aborted", "Bad print record", "Print driver error", "Windows error during printing", "Memory error during printing", "Print dialog error", "Generic print error", "Invalid device refnum", "Device not found", "Device parameter error", "Device unit error", "Cannot open device", "Device call aborted", "Generic error", "Cancelled by user", "Object ID too low", "Object ID too high", "Object not in heap", "Unknown heap", "Unknown object (invalid DefProc)", "Unknown object (DefProc not in table)", "Message out of range", "Invalid (null) method", "Unknown message", "Manager call not supported", "Bad address", "Network operation in progress", "Network operation timed out", "Connection is busy", "Network attribute not supported", "Network error", "Address in use", "System out of memory", "Connection aborted", "Connection refused", "Not connected", "Already connected", "Connection closed", "Initialization error (interapplication manager)", "Bad occurrence", "Wait on unbound occurrence handler", "Occurrence queue overflow", "Datalog type conflict", "Unused", "Unrecognized type (interapplication manager)", "Memory corrupt", "Failed to make temporary DLL", "Old CIN version", "Drag socket not found", "Failed to load drop-object", "Failed to register OLE object", "Failed to release OLE object", "Format specifier type mismatch", "Unknown format specifier", "Too few format specifiers", "Too many format specifiers", "Scan failed", "Newer CIN version", "Error converting to variant", "Runtime menu error", "Password tampered", "Variant attribute not found", "Incompatible variant data type", "Event data is not available", "Event Store is not present", "Occurrence is not found", "Event Queue is not created", "Event info is not available", "Refnum passed is NULL", "Error retrieving Class GUID", "Error retrieving CoClass GUID", "Error retrieving TypeLib GUID.", "Bad built application magic bytes.", "Specific driver is different from the specific driver associated with the Logical Name.", "There is no session opened to the class driver.", "Max Error", "MAX - Error with config objects", "MAX - Error loading configuration", "MAX - Group not supported"]
            # "Current State"
            # "Do not delete, rename, or modify this frame.\n(this is used to capture unhandled states and typos)"
            # "Handle mistyped state name (developer tool)"
            n234 = Format Into String(format string="Software Exception: Unhandled State \"%s\"." ("message"), error in=w404, w399) -> (resulting string=w407:string, error out=w406:errorcluster)  [unwired: 1 in]
            n235 = call <vilib>:"Error Cluster From Error Code.vi"("show call chain? (False)"=TRUE, "error in (no error)"=w406, "error message (\"\")"=w407, "error code (0)"=w408) -> ("error out"=w405:errorcluster)  [unwired: 5 in]
            n236 = call <vilib>:"Add State(s) to Queue__jki_lib_state_machine.vi"("State(s) in (\"\")"=w403) -> ("States Out"=w402:string)  [unwired: 14 in]
          }
          frame "Initialize Core Data" {
            # "Do not delete, rename, or modify this frame.\n(this is used to determine panel behavior on exit)"
            # "originally closed?"
            # "exe?"
            # "If panel starts closed or is an EXE, then close it when we exit"
            n237 = property class="VI"() -> ("Front Panel.Open"=w417:bool)  [unwired: 2 in, 2 out]
            n238 = property class="App"() -> ("App.Kind"=w416:T41)  [unwired: 2 in, 2 out]
            n239 = control-ref of="Current VI Reference"() -> (w410:refnum<vi>)
            n240 = Not(x=w417) -> (.not. x?=w414:bool)
            n241 = Equal?(x=w416, y=T41."Run Time System" ("Application:Kind")) -> (x = y?=w413:bool)
            n242 = Or(x=w414, y=w413) -> (x .or. y?=w411:bool)
            n243 = Bundle By Name(cluster=w412, "Core.Current VI Reference"=w410, "Core.Close Panel on Exit?"=w411) -> (w419:T48)
            n244 = call <vilib>:"Add State(s) to Queue__jki_lib_state_machine.vi"("State(s) in (\"\")"=w421) -> ("States Out"=w420:string)  [unwired: 14 in]
          }
          frame "Error Handler" {
            w432 = i32[] [-1950679035, -1950678943]  # Error Codes to Filter
            # "Unhandled Error -- Display it"
            # "Handle any errors here.\nYou can also output any states to clean-up after errors occur"
            # "Clear error"
            n245 = call-poly <userlib>:"Filter Error Codes__ogtk.vi"("Error In"=w433, "Error Codes to Filter"=w432) -> ("Error Out"=w434:errorcluster, "Filtered Error Details"=w431:T53)  [unwired: 7 in, 1 out]
            n246 = Unbundle(w431) -> ("code"=w429:i32, "source"=w430:string)
            n247 = Get Date/Time In Seconds() -> (seconds since 1Jan1904=w428:timestamp)
            n248 = Unbundle By Name(w424) -> ("Error Log"=w426:T34)
            n249 = Bundle By Name(cluster=T42 {"time"=timestamp(0 s since 1904-01-01), "code"=0, "source"=""} ("output cluster"), "time"=w428, "code"=w429, "source"=w430) -> (w425:T42)
            n250 = Build Array (concatenate)(w426, w425) -> (w422:T34)
            "Error List" <- w422
            n251 = Bundle By Name(cluster=w424, "Error Log"=w422) -> (w423:T48)
            n252 = call <vilib>:"General Error Handler.vi"("error in (no error)"=w434) -> ()  [unwired: 10 in, 5 out]
            n253 = call <vilib>:"Add State(s) to Queue__jki_lib_state_machine.vi"("State(s) in Front (\"\")"="/* Post Error States", "State(s) in (\"\")"=w438) -> ("States Out"=w437:string)  [unwired: 13 in]
          }
          frame "Exit" {
            # "Do not put any code in this frame.\n(No errors that occur here will be handled.)"
            n254 = call <vilib>:"Add State(s) to Queue__jki_lib_state_machine.vi"("State(s) in (\"\")"=w443) -> ("States Out"=w442:string)  [unwired: 14 in]
          }
          frame "---------- Data ----------" {
            # "Do not put any code in this frame.\n(It is a separator no-op. You can make a copy of this frame to create a new Data frame)"
            n255 = call <vilib>:"Add State(s) to Queue__jki_lib_state_machine.vi"("State(s) in (\"\")"=w447) -> ("States Out"=w446:string)  [unwired: 14 in]
          }
          frame "Data: Initialize" {
            w448 = T34 []  # Error Log
            w450 = TRUE  # sentinel
            w451 = T47 {"Comms"="", "Device ID"=[], "Comms Layer"=enum."Ethernet TCP/IP", "Command"="", "Query reference"=refnum}  # Mercury IPS Ref
            w452 = T52 {"Comms"="", "Device ID"=[], "Comms Layer"=enum."Ethernet TCP/IP", "Command"="", "Query reference"=refnum}  # Mercury ITC Ref
            w453 = T54 {"Current VI Reference"=refnum, "Close Panel on Exit?"=FALSE}  # Core
            # "do not delete - used by framework"
            # "Expand Bundle to add new data elements to shift register data."
            # "Add new data here."
            # "Data names and types of shift register data are defined by this bundle."
            # "Initialize the shift-register data, here.\n(data names are defined by what you wire into the bundle function)"
            n256 = Bundle("Core"=w453, "Mercury ITC Ref"=w452, "Mercury IPS Ref"=w451, "sentinel"=w450, "Error Log"=w448) -> (w454:T48)  [unwired: 1 in]
            n257 = call <vilib>:"Add State(s) to Queue__jki_lib_state_machine.vi"("State(s) in (\"\")"=w456) -> ("States Out"=w455:string)  [unwired: 14 in]
          }
          frame "Data: Cleanup" {
            # "Cleanup any data and references, here.\n(this is called automatically, by the Macro: Exit)"
            n258 = Unbundle By Name(w457) -> ("Core.Current VI Reference"=w460:refnum<vi>)
            n259 = Close Reference(reference=w460, error in (no error)=w459) -> (error out=w458:errorcluster)
            n260 = call <vilib>:"Add State(s) to Queue__jki_lib_state_machine.vi"("State(s) in (\"\")"=w462) -> ("States Out"=w461:string)  [unwired: 14 in]
          }
          frame "---------- UI ----------" {
            # "Do not put any code in this frame.\n(It is a separator no-op. You can make a copy of this frame to create a new UI frame)"
            n261 = call <vilib>:"Add State(s) to Queue__jki_lib_state_machine.vi"("State(s) in (\"\")"=w466) -> ("States Out"=w465:string)  [unwired: 14 in]
          }
          frame "UI: Initialize" {
            w473 = FALSE
            # "start in local mode"
            # "Initialize the User Interface, here.\n(this is called automatically, by the Macro: Init)"
            n262 = disable-structure shown="Enabled" {
              frame Disabled {
                n263 = Open VI Reference(vi path=path "") -> ()  [unwired: 5 in, 2 out]
                n264 = call "MNK_Dashboard_v2.vi"() -> ()  [unwired: 12 in]
              }
              frame Enabled {
              }
            }
            n265 = Open Application Reference(8:w468) -> (0:w470:errorcluster, 3:w471:refnum<vi>)  [unwired: 3 in]
            n266 = property class="App"(reference=w471, error in=w470, "WebSrvr.Active"=TRUE ("Web Server:Server Active")) -> (error out=w467:errorcluster)  [unwired: 1 out]
            n267 = call <vilib>:"Add State(s) to Queue__jki_lib_state_machine.vi"("State(s) in (\"\")"=w478) -> ("States Out"=w477:string)  [unwired: 14 in]
            n268 = local write "Remote Mode"(w473) -> ()
            n269 = call <userlib>:"FGV_PSP - Mercury Remote.vi"("error in"=w467, "Function"=enum16{"write", "read"}."write", "Remote"=w473) -> ("error out"=w472:errorcluster)  [unwired: 3 in, 1 out]
            "Magnet Status 2" <- "" ("Magnet Status 2")
          }
          frame "UI: Cursor Set" {
            # "Argument"
            # "Set and Unset Cursor Busy.\n(Usage: \"UI: Cursor Set >> Busy|Idle\")"
            n270 = case shown="\"Idle\", Default" w480 {
              tunnel: w482 -> [w487 w489]
              tunnel: [w486 w488] -> w481
              frame "Idle", Default {
                n271 = call <vilib>:"Unset Busy.vi"("error in (no error)"=w487) -> ("error out"=w486:errorcluster)  [unwired: 10 in]
              }
              frame "Busy" {
                n272 = call <vilib>:"Set Busy.vi"("error in (no error)"=w489) -> ("error out"=w488:errorcluster)  [unwired: 9 in, 1 out]
              }
            }
            n273 = call <vilib>:"Add State(s) to Queue__jki_lib_state_machine.vi"("State(s) in (\"\")"=w485) -> ("States Out"=w484:string)  [unwired: 14 in]
          }
          frame "UI: Front Panel State" {
            # "Argument"
            # "Set Front Panel Open or Closed\n(Usage: \"UI: Front Panel State >> Open|Close\")"
            n274 = Unbundle By Name(w492) -> ("Core.Current VI Reference"=w491:refnum<vi>)
            n275 = case shown="\"Open\", Default" w490 {
              tunnel: w494 -> [w500 w513]
              tunnel: [w502 w514] -> w493
              tunnel: w491 -> [w501 w511]
              frame "Open", Default {
                n276 = property class="VI"(reference=w501, error in=w500) -> (reference out=w498:refnum<vi>, error out=w499:errorcluster, "Front Panel.Open"=w497:bool)
                n277 = case shown="True" w497 {
                  tunnel: [w505 w508] -> w502
                  tunnel: w499 -> [w504 w508]
                  tunnel: w498 -> [w503 _]
                  frame False {
                    n278 = invoke class="VI" method="FP.Open"(reference=w503, error in=w504, "Activate"=TRUE, "State"=T43."Standard") -> (error out=w505:errorcluster)  [unwired: 1 in, 4 out]
                  }
                  frame True {
                  }
                }
              }
              frame "Close" {
                n279 = property class="VI"(reference=w511, error in=w513) -> (reference out=w510:refnum<vi>, error out=w512:errorcluster, "Front Panel.Open"=w509:bool)
                n280 = case shown="True" w509 {
                  tunnel: [w515 w518] -> w514
                  tunnel: w512 -> [w515 w517]
                  tunnel: w510 -> [_ w516]
                  frame False {
                  }
                  frame True {
                    n281 = invoke class="VI" method="FP.Close"(reference=w516, error in=w517) -> (error out=w518:errorcluster)  [unwired: 1 in, 2 out]
                  }
                }
              }
            }
            n282 = call <vilib>:"Add State(s) to Queue__jki_lib_state_machine.vi"("State(s) in (\"\")"=w496) -> ("States Out"=w495:string)  [unwired: 14 in]
          }
          frame "---------- Macro ----------" {
            # "Do not put any code in this frame.\n(It is a separator no-op. You can make a copy of this frame to create a new Macro frame)"
            n283 = call <vilib>:"Add State(s) to Queue__jki_lib_state_machine.vi"("State(s) in (\"\")"=w522) -> ("States Out"=w521:string)  [unwired: 14 in]
          }
          frame "Macro: Initialize" {
            w523 = "Data: Initialize\nInitialize Core Data\nUI: Initialize\nUI: Front Panel State >> Open\nMercury: Initialize"  # Data: Initialize Initialize Core Data UI: Initialize UI: Front Panel State >> Open Mercury: Initialize
            # "Initialization Macro\n(This is called once, when the VI starts)"
            n284 = call <vilib>:"Add State(s) to Queue__jki_lib_state_machine.vi"("State(s) in Front (\"\")"=w523, "State(s) in (\"\")"=w527) -> ("States Out"=w526:string)  [unwired: 13 in]
          }
          frame "Macro: Exit" {
            # "Exit Macro\n(This is called once, when the VI exits)"
            n285 = Unbundle By Name(w540) -> ("Core.Close Panel on Exit?"=w539:bool, "Mercury ITC Ref"=w532:T52, "Mercury IPS Ref"=w531:T47)
            n286 = call <instrlib>:"Close.vi"("error in (no error)"=w530, "Mercury Reference"=w531) -> ("error out"=w529:errorcluster)  [unwired: 9 out]
            n287 = call <instrlib>:"Close.vi"("error in (no error)"=w529, "Mercury Reference"=w532) -> ("error out"=w533:errorcluster)  [unwired: 9 out]
            n288 = call <vilib>:"Simple Error Handler.vi"("error in (no error)"=w533) -> ("error out"=w528:errorcluster)  [unwired: 1 in, 7 out]
            n289 = Select(t="UI: Front Panel State >> Close", s=w539, f="") -> (s? t:f=w536:string)
            n290 = call <vilib>:"Add State(s) to Queue__jki_lib_state_machine.vi"("State(s) in (\"\")"=w536, "State(s) at Back (\"\")"="Data: Cleanup\nExit") -> ("States Out"=w534:string)  [unwired: 13 in]
            n291 = call <vilib>:"Add State(s) to Queue__jki_lib_state_machine.vi"("State(s) in Front (\"\")"=w534, "State(s) in (\"\")"=w542) -> ("States Out"=w541:string)  [unwired: 13 in]
          }
          frame "---------- New Category ----------" {
            n292 = call <vilib>:"Add State(s) to Queue__jki_lib_state_machine.vi"("State(s) in (\"\")"=w546) -> ("States Out"=w545:string)  [unwired: 14 in]
          }
          frame "Mercury: Initialize" {
            w555 = Comms_Transport_Layer."Ethernet TCP/IP" ("Comms Layer")
            n293 = call-poly <instrlib>:"Open.vi"("Clear Previous Connections (False)"=TRUE ("Clear Previous Connections (True)"), "ID Query (True)"=TRUE, "IP Address"="ITC IP Address", "error in (no error)"=w556, "Comms Layer"=w555) -> ("error out"=w549:errorcluster, "# of Instruments"=→"# of Instruments":i32, "Serial Number(s)"=→"Serial Number(s)":string[], "Mercury Reference Out"=w550:T47, "S/W Version(s)"=→"S/W Version(s)":string[])  [unwired: 2 in]
            n294 = call-poly <instrlib>:"Open.vi"("Clear Previous Connections (False)"=FALSE ("Clear Previous Connections (True)"), "ID Query (True)"=TRUE, "IP Address"="IPS IP Address", "error in (no error)"=w549, "Comms Layer"=w555) -> ("error out"=w548:errorcluster, "# of Instruments"=→"# of Instruments 2":i32, "Serial Number(s)"=→"Serial Number(s) 2":string[], "Mercury Reference Out"=w547:T47, "S/W Version(s)"=→"S/W Version(s) 2":string[])  [unwired: 2 in]
            n295 = Bundle By Name(cluster=w564, "Mercury ITC Ref"=w550, "Mercury IPS Ref"=w547) -> (w563:T48)
            n296 = call <vilib>:"Add State(s) to Queue__jki_lib_state_machine.vi"("State(s) in (\"\")"=w569, "State(s) at Back (\"\")"="Mercury: Query ITC: System\nMercury: Query IPS: System\nMercury: Query ITC: Temperature\nMercury: Query ITC: Heater\nMercury: Query ITC: Aux\nMercury: Query ITC: Pressure\nMercury: Query IPS: LVL\nMercury: Query IPS: Temperature\nMercury: Query IPS: Magnet" ("State(s) at Back (\"\")")) -> ("States Out"=w568:string)  [unwired: 13 in]
          }
          frame "Mercury: Query ITC: System" {
            n297 = Unbundle By Name(w611) -> ("Mercury ITC Ref"=w571:T52)
            n298 = call-poly <instrlib>:"Configuration (Read).vi"("error in"=w575, "Mercury Reference In"=w571) -> ("error out"=w607:errorcluster, "Devices"=→"ITC Devices":string[], "Mercury Reference Out"=w608:T47)  [unwired: 1 in, 6 out]
            n299 = call-poly <instrlib>:"Configuration (Read).vi"("error in"=w607, "Mercury Reference In"=w608) -> ("error out"=w600:errorcluster, "Automatic Dimming"=→"Automatic Dimming":string, "Mercury Reference Out"=w601:T47)  [unwired: 1 in, 6 out]
            n300 = call-poly <instrlib>:"Configuration (Read).vi"("error in"=w600, "Mercury Reference In"=w601) -> ("error out"=w603:errorcluster, "Dimming Time"=→"Dimming Time":string, "Mercury Reference Out"=w602:T47)  [unwired: 1 in, 6 out]
            n301 = call-poly <instrlib>:"Configuration (Read).vi"("error in"=w603, "Mercury Reference In"=w602) -> ("error out"=w609:errorcluster, "Display Brightness"=→"Display Brightness":string, "Mercury Reference Out"=w610:T47)  [unwired: 1 in, 6 out]
            n302 = call-poly <instrlib>:"Configuration (Read).vi"("error in"=w609, "Mercury Reference In"=w610) -> ("error out"=w594:errorcluster, "Date"=→"Date":string, "Mercury Reference Out"=w593:T47)  [unwired: 1 in, 6 out]
            n303 = call-poly <instrlib>:"Configuration (Read).vi"("error in"=w594, "Mercury Reference In"=w593) -> ("error out"=w596:errorcluster, "Time"=→"Time":string, "Mercury Reference Out"=w595:T47)  [unwired: 1 in, 6 out]
            n304 = call-poly <instrlib>:"Configuration (Read).vi"("error in"=w596, "Mercury Reference In"=w595) -> ("error out"=w574:errorcluster, "time stamp"=→"time stamp":timestamp, "Mercury Reference Out"=w572:T47)  [unwired: 1 in, 6 out]
            n305 = call-poly <instrlib>:"Configuration (Read).vi"("error in"=w574, "Mercury Reference In"=w572) -> ("error out"=w592:errorcluster, "Hardware Version"=→"Hardware Version":string, "Mercury Reference Out"=w591:T47)  [unwired: 1 in, 6 out]
            n306 = call-poly <instrlib>:"Configuration (Read).vi"("error in"=w592, "Mercury Reference In"=w591) -> ("error out"=w590:errorcluster, "Firmware Version"=→"Firmware Version":string, "Mercury Reference Out"=w589:T47)  [unwired: 1 in, 6 out]
            n307 = call-poly <instrlib>:"Configuration (Read).vi"("error in"=w590, "Mercury Reference In"=w589) -> ("error out"=w577:errorcluster, "Serial Number"=→"Serial Number":string, "Mercury Reference Out"=w576:T47)  [unwired: 1 in, 6 out]
            n308 = call-poly <instrlib>:"Configuration (Read).vi"("error in"=w577, "Mercury Reference In"=w576) -> ("error out"=w583:errorcluster, "Free Space"=→"Free Space":i32, "Mercury Reference Out"=w582:T47)  [unwired: 1 in, 6 out]
            n309 = call-poly <instrlib>:"Configuration (Read).vi"("error in"=w583, "Mercury Reference In"=w582) -> ("error out"=w579:errorcluster, "Mode"=→"String":T55, "Mercury Reference Out"=w580:T47)  [unwired: 1 in, 6 out]
            n310 = Get Date/Time In Seconds() -> (seconds since 1Jan1904=w588:timestamp)
            n311 = call-poly <instrlib>:"Configuration (Set).vi"("error in"=w579, "time stamp"=w588, "Mercury Reference In"=w580) -> ("error out"=w573:errorcluster, "Response"=→"Set Date Response":T40)  [unwired: 1 in, 6 out]
            n312 = call <vilib>:"Add State(s) to Queue__jki_lib_state_machine.vi"("State(s) in (\"\")"=w613) -> ("States Out"=w612:string)  [unwired: 14 in]
          }
          frame "Mercury: Query ITC: Temperature" {
            # "Temperature"
            n313 = Unbundle By Name(w658) -> ("Mercury ITC Ref"=w615:T52)
            n314 = local read "ITC Devices"() -> (w614:string[])
            n315 = Index Array(array=w614, index=3) -> (element=w616:string)
            n316 = call-poly <instrlib>:"Open.vi"("error in (no error)"=w621, "Device Identifier"=w616, "Mercury Reference In"=w615) -> ("error out"=w633:errorcluster, "Mercury Reference Out"=w634:T47)  [unwired: 7 out]
            n317 = call-poly <instrlib>:"Configuration (Read).vi"("error in"=w633, "Mercury Reference In"=w634) -> ("error out"=w625:errorcluster, "Serial Number"=→"Temp S/N":string, "Mercury Reference Out"=w624:T47)  [unwired: 1 in, 6 out]
            n318 = call-poly <instrlib>:"Configuration (Read).vi"("error in"=w625, "Mercury Reference In"=w624) -> ("error out"=w627:errorcluster, "Nickname"=→"T Nickname":string, "Mercury Reference Out"=w626:T47)  [unwired: 1 in, 6 out]
            n319 = call-poly <instrlib>:"Configuration (Read).vi"("error in"=w627, "Mercury Reference In"=w626) -> ("error out"=w630:errorcluster, "Unit"=→"Unit":T3, "Excitation Magnitude"=→"Excitation Magnitude":dbl, "Mercury Reference Out"=w629:T47)  [unwired: 1 in, 5 out]
            n320 = call-poly <instrlib>:"Configuration (Read).vi"("error in"=w630, "Mercury Reference In"=w629) -> ("error out"=w619:errorcluster, "Sensor Type"=→"Sensor Type":T6, "Mercury Reference Out"=w617:T47)  [unwired: 1 in, 6 out]
            n321 = call-poly <instrlib>:"Configuration (Read).vi"("error in"=w619, "Mercury Reference In"=w617) -> ("error out"=w636:errorcluster, "Excitation Type"=→"Excitation Type":T8, "Mercury Reference Out"=w637:T47)  [unwired: 1 in, 6 out]
            n322 = call-poly <instrlib>:"Configuration (Read).vi"("error in"=w636, "Mercury Reference In"=w637) -> ("error out"=w638:errorcluster, "Unit"=→"H Unit":T3, "Hot Limit"=→"Hot Limit":dbl, "Mercury Reference Out"=w639:T47)  [unwired: 1 in, 5 out]
            n323 = call-poly <instrlib>:"Configuration (Read).vi"("error in"=w638, "Mercury Reference In"=w639) -> ("error out"=w645:errorcluster, "Unit"=→"C Unit":T3, "Cold Limit"=→"Cold Limit":dbl, "Mercury Reference Out"=w644:T47)  [unwired: 1 in, 5 out]
            n324 = call-poly <instrlib>:"Signals (Read).vi"("error in"=w645, "Mercury Reference In"=w644) -> ("error out"=w649:errorcluster, "Unit"=→"V Unit":T3, "Voltage"=→"Voltage":dbl, "Mercury Reference Out"=w648:T47)  [unwired: 1 in, 5 out]
            n325 = call-poly <instrlib>:"Signals (Read).vi"("error in"=w649, "Mercury Reference In"=w648) -> ("error out"=w650:errorcluster, "Unit"=→"T Unit":T3, "Temperature"=→"Temperature":dbl, "Mercury Reference Out"=w653:T47)  [unwired: 1 in, 5 out]
            n326 = call-poly <instrlib>:"Configuration (Read).vi"("error in"=w650, "Mercury Reference In"=w653) -> ("error out"=w656:errorcluster, "Device Details"=→"Temperature Device Settings":T4, "Mercury Reference Out"=w655:T47)  [unwired: 1 in, 6 out]
            n327 = call-poly <instrlib>:"Configuration (Read).vi"("error in"=w656, "Mercury Reference In"=w655) -> ("error out"=w620:errorcluster, "Loop Details"=→"T Loop Details":T11)  [unwired: 1 in, 7 out]
            n328 = call <vilib>:"Add State(s) to Queue__jki_lib_state_machine.vi"("State(s) in (\"\")"=w659) -> ("States Out"=w660:string)  [unwired: 14 in]
          }
          frame "Mercury: Query ITC: Heater" {
            # "Heater"
            n329 = Unbundle By Name(w665) -> ("Mercury ITC Ref"=w664:T52)
            n330 = local read "ITC Devices"() -> (w666:string[])
            n331 = Index Array(array=w666, index=2) -> (element=w661:string)
            n332 = call-poly <instrlib>:"Open.vi"("error in (no error)"=w668, "Device Identifier"=w661, "Mercury Reference In"=w664) -> ("error out"=w671:errorcluster, "Mercury Reference Out"=w670:T47)  [unwired: 7 out]
            n333 = call-poly <instrlib>:"Configuration (Read).vi"("error in"=w671, "Mercury Reference In"=w670) -> ("error out"=w678:errorcluster, "Device Details"=→"Heater Device Settings":T13, "Mercury Reference Out"=w677:T47)  [unwired: 1 in, 6 out]
            n334 = call-poly <instrlib>:"Configuration (Read).vi"("error in"=w678, "Mercury Reference In"=w677) -> ("error out"=w680:errorcluster, "Nickname"=→"Htr Nickname":string, "Mercury Reference Out"=w679:T47)  [unwired: 1 in, 6 out]
            n335 = call-poly <instrlib>:"Configuration (Read).vi"("error in"=w680, "Mercury Reference In"=w679) -> ("error out"=w673:errorcluster, "Serial Number"=→"Htr S/N":string, "Mercury Reference Out"=w672:T47)  [unwired: 1 in, 6 out]
            n336 = call-poly <instrlib>:"Configuration (Read).vi"("error in"=w673, "Mercury Reference In"=w672) -> ("error out"=w669:errorcluster, "Unit"=→"Volt Unit":T3, "Voltage Limit"=→"Htr Voltage Limit":dbl, "Mercury Reference Out"=w663:T47)  [unwired: 1 in, 5 out]
            n337 = call-poly <instrlib>:"Configuration (Read).vi"("error in"=w669, "Mercury Reference In"=w663) -> ("error out"=w683:errorcluster, "Unit"=→"Res Unit":T3, "Nominal Resistance"=→"Htr Resistance":dbl, "Mercury Reference Out"=w684:T47)  [unwired: 1 in, 5 out]
            n338 = call-poly <instrlib>:"Configuration (Read).vi"("error in"=w683, "Mercury Reference In"=w684) -> ("error out"=w690:errorcluster, "Unit"=→"Power Unit":T3, "Maximum Power"=→"Maximum Power":dbl, "Mercury Reference Out"=w689:T47)  [unwired: 1 in, 5 out]
            n339 = call-poly <instrlib>:"Signals (Read).vi"("error in"=w690, "Mercury Reference In"=w689) -> ("error out"=w692:errorcluster, "Unit"=→"Htr V Unit":T3, "Voltage"=→"Htr Voltage":dbl, "Mercury Reference Out"=w691:T47)  [unwired: 1 in, 5 out]
            n340 = call-poly <instrlib>:"Signals (Read).vi"("error in"=w692, "Mercury Reference In"=w691) -> ("error out"=w694:errorcluster, "Unit"=→"Htr P Unit":T3, "Power"=→"Htr Power":dbl, "Mercury Reference Out"=w693:T47)  [unwired: 1 in, 5 out]
            n341 = call-poly <instrlib>:"Signals (Read).vi"("error in"=w694, "Mercury Reference In"=w693) -> ("error out"=w662:errorcluster, "Unit"=→"Htr C Unit":T3, "Current"=→"Htr Current":dbl)  [unwired: 1 in, 6 out]
            n342 = call <vilib>:"Add State(s) to Queue__jki_lib_state_machine.vi"("State(s) in (\"\")"=w701) -> ("States Out"=w702:string)  [unwired: 14 in]
          }
          frame "Mercury: Query ITC: Aux" {
            # "Auxiliary"
            n343 = Unbundle By Name(w708) -> ("Mercury ITC Ref"=w703:T52)
            n344 = local read "ITC Devices"() -> (w706:string[])
            n345 = Index Array(array=w706, index=0) -> (element=w704:string)
            n346 = call-poly <instrlib>:"Open.vi"("error in (no error)"=w710, "Device Identifier"=w704, "Mercury Reference In"=w703) -> ("error out"=w730:errorcluster, "Mercury Reference Out"=w731:T47)  [unwired: 7 out]
            n347 = call-poly <instrlib>:"Configuration (Read).vi"("error in"=w730, "Mercury Reference In"=w731) -> ("error out"=w734:errorcluster, "Auxiliary Device Details"=→"Auxiliary Device Details":T21, "Mercury Reference Out"=w733:T47)  [unwired: 1 in, 6 out]
            n348 = call-poly <instrlib>:"Configuration (Read).vi"("error in"=w734, "Mercury Reference In"=w733) -> ("error out"=w737:errorcluster, "Serial Number"=→"Aux S/N":string, "Mercury Reference Out"=w736:T47)  [unwired: 1 in, 6 out]
            n349 = call-poly <instrlib>:"Configuration (Read).vi"("error in"=w737, "Mercury Reference In"=w736) -> ("error out"=w739:errorcluster, "Unit"=→"Unit 2":T3, "Min Flow"=→"Min Flow":dbl, "Mercury Reference Out"=w738:T47)  [unwired: 1 in, 5 out]
            n350 = call-poly <instrlib>:"Configuration (Read).vi"("error in"=w739, "Mercury Reference In"=w738) -> ("error out"=w741:errorcluster, "Unit"=→"Unit 3":T3, "Scaling Factor"=→"Scaling Factor":dbl, "Mercury Reference Out"=w740:T47)  [unwired: 1 in, 5 out]
            n351 = call-poly <instrlib>:"Configuration (Read).vi"("error in"=w741, "Mercury Reference In"=w740) -> ("error out"=w709:errorcluster, "Unit"=→"Unit 4":T3, "Temp Err"=→"Temp Err":dbl, "Mercury Reference Out"=w705:T47)  [unwired: 1 in, 5 out]
            n352 = call-poly <instrlib>:"Configuration (Read).vi"("error in"=w709, "Mercury Reference In"=w705) -> ("error out"=w713:errorcluster, "Unit"=→"Unit 5":T3, "Temp V Err"=→"Temp V Err":dbl, "Mercury Reference Out"=w712:T47)  [unwired: 1 in, 5 out]
            n353 = call-poly <instrlib>:"Configuration (Read).vi"("error in"=w713, "Mercury Reference In"=w712) -> ("error out"=w715:errorcluster, "Unit"=→"Unit 6":T3, "Gear"=→"Gear":u32, "Mercury Reference Out"=w714:T47)  [unwired: 1 in, 5 out]
            n354 = call-poly <instrlib>:"Configuration (Read).vi"("error in"=w715, "Mercury Reference In"=w714) -> ("error out"=w723:errorcluster, "Unit"=→"Unit 7":T3, "Speed"=→"Speed":u32, "Mercury Reference Out"=w722:T47)  [unwired: 1 in, 5 out]
            n355 = call-poly <instrlib>:"Signals (Read).vi"("error in"=w723, "Mercury Reference In"=w722) -> ("error out"=w725:errorcluster, "Unit"=→"Unit":T3, "Position"=→"Position":u32, "Mercury Reference Out"=w724:T47)  [unwired: 1 in, 5 out]
            n356 = call-poly <instrlib>:"Signals (Read).vi"("error in"=w725, "Mercury Reference In"=w724) -> ("error out"=w711:errorcluster, "Unit"=→"Unit":T3, "% Open"=→"% Open":dbl)  [unwired: 1 in, 6 out]
            n357 = call <vilib>:"Add State(s) to Queue__jki_lib_state_machine.vi"("State(s) in (\"\")"=w748) -> ("States Out"=w749:string)  [unwired: 14 in]
          }
          frame "Mercury: Query ITC: Pressure" {
            # "Pressure"
            n358 = Unbundle By Name(w755) -> ("Mercury ITC Ref"=w752:T52)
            n359 = local read "ITC Devices"() -> (w754:string[])
            n360 = Index Array(array=w754, index=1) -> (element=w751:string)
            n361 = call-poly <instrlib>:"Open.vi"("error in (no error)"=w750, "Device Identifier"=w751, "Mercury Reference In"=w752) -> ("error out"=w758:errorcluster, "Mercury Reference Out"=w759:T47)  [unwired: 7 out]
            n362 = call-poly <instrlib>:"Configuration (Read).vi"("error in"=w758, "Mercury Reference In"=w759) -> ("error out"=w760:errorcluster, "Device Details"=→"Pressure Device":T15, "Mercury Reference Out"=w761:T47)  [unwired: 1 in, 6 out]
            n363 = call-poly <instrlib>:"Configuration (Read).vi"("error in"=w760, "Mercury Reference In"=w761) -> ("error out"=w765:errorcluster, "Nickname"=→"Nickname":string, "Mercury Reference Out"=w766:T47)  [unwired: 1 in, 6 out]
            n364 = call-poly <instrlib>:"Signals (Read).vi"("error in"=w765, "Mercury Reference In"=w766) -> ("error out"=w763:errorcluster, "Current"=→"Current":dbl, "Mercury Reference Out"=w764:T47)  [unwired: 1 in, 6 out]
            n365 = call-poly <instrlib>:"Signals (Read).vi"("error in"=w763, "Mercury Reference In"=w764) -> ("error out"=w756:errorcluster, "Voltage"=→"Voltage":dbl)  [unwired: 1 in, 7 out]
            n366 = call <vilib>:"Add State(s) to Queue__jki_lib_state_machine.vi"("State(s) in (\"\")"=w769) -> ("States Out"=w770:string)  [unwired: 14 in]
          }
          frame "Mercury: Query IPS: System" {
            # "Your code here.\n(You can make a copy of, or modify, this frame)"
            n367 = Unbundle By Name(w812) -> ("Mercury IPS Ref"=w773:T47)
            n368 = call-poly <instrlib>:"Configuration (Read).vi"("error in"=w778, "Mercury Reference In"=w773) -> ("error out"=w798:errorcluster, "Devices"=→"IPS Devices":string[], "Mercury Reference Out"=w797:T47)  [unwired: 1 in, 6 out]
            n369 = call-poly <instrlib>:"Configuration (Read).vi"("error in"=w798, "Mercury Reference In"=w797) -> ("error out"=w802:errorcluster, "Automatic Dimming"=→"Automatic Dimming 2":string, "Mercury Reference Out"=w801:T47)  [unwired: 1 in, 6 out]
            n370 = call-poly <instrlib>:"Configuration (Read).vi"("error in"=w802, "Mercury Reference In"=w801) -> ("error out"=w799:errorcluster, "Dimming Time"=→"Dimming Time 2":string, "Mercury Reference Out"=w800:T47)  [unwired: 1 in, 6 out]
            n371 = call-poly <instrlib>:"Configuration (Read).vi"("error in"=w799, "Mercury Reference In"=w800) -> ("error out"=w796:errorcluster, "Display Brightness"=→"Display Brightness 2":string, "Mercury Reference Out"=w795:T47)  [unwired: 1 in, 6 out]
            n372 = call-poly <instrlib>:"Configuration (Read).vi"("error in"=w796, "Mercury Reference In"=w795) -> ("error out"=w805:errorcluster, "Date"=→"Date 2":string, "Mercury Reference Out"=w806:T47)  [unwired: 1 in, 6 out]
            n373 = call-poly <instrlib>:"Configuration (Read).vi"("error in"=w805, "Mercury Reference In"=w806) -> ("error out"=w803:errorcluster, "Time"=→"Time 2":string, "Mercury Reference Out"=w804:T47)  [unwired: 1 in, 6 out]
            n374 = call-poly <instrlib>:"Configuration (Read).vi"("error in"=w803, "Mercury Reference In"=w804) -> ("error out"=w777:errorcluster, "time stamp"=→"time stamp 2":timestamp, "Mercury Reference Out"=w774:T47)  [unwired: 1 in, 6 out]
            n375 = call-poly <instrlib>:"Configuration (Read).vi"("error in"=w777, "Mercury Reference In"=w774) -> ("error out"=w779:errorcluster, "Hardware Version"=→"Hardware Version 2":string, "Mercury Reference Out"=w780:T47)  [unwired: 1 in, 6 out]
            n376 = call-poly <instrlib>:"Configuration (Read).vi"("error in"=w779, "Mercury Reference In"=w780) -> ("error out"=w781:errorcluster, "Firmware Version"=→"Firmware Version 2":string, "Mercury Reference Out"=w782:T47)  [unwired: 1 in, 6 out]
            n377 = call-poly <instrlib>:"Configuration (Read).vi"("error in"=w781, "Mercury Reference In"=w782) -> ("error out"=w787:errorcluster, "Serial Number"=→"Serial Number 2":string, "Mercury Reference Out"=w788:T47)  [unwired: 1 in, 6 out]
            n378 = call-poly <instrlib>:"Configuration (Read).vi"("error in"=w787, "Mercury Reference In"=w788) -> ("error out"=w783:errorcluster, "Free Space"=→"Free Space 2":i32, "Mercury Reference Out"=w784:T47)  [unwired: 1 in, 6 out]
            n379 = call-poly <instrlib>:"Configuration (Read).vi"("error in"=w783, "Mercury Reference In"=w784) -> ("error out"=w786:errorcluster, "Mode"=→"String 2":T55, "Mercury Reference Out"=w785:T47)  [unwired: 1 in, 6 out]
            n380 = Get Date/Time In Seconds() -> (seconds since 1Jan1904=w794:timestamp)
            n381 = call-poly <instrlib>:"Configuration (Set).vi"("error in"=w786, "time stamp"=w794, "Mercury Reference In"=w785) -> ("error out"=w776:errorcluster, "Response"=→"Set Date Response 2":T40)  [unwired: 1 in, 6 out]
            n382 = call <vilib>:"Add State(s) to Queue__jki_lib_state_machine.vi"("State(s) in (\"\")"=w814) -> ("States Out"=w813:string)  [unwired: 14 in]
          }
          frame "Mercury: Query IPS: LVL" {
            # "Level"
            n383 = Unbundle By Name(w854) -> ("Mercury IPS Ref"=w817:T47)
            n384 = local read "IPS Devices"() -> (w853:string[])
            n385 = Index Array(array=w853, index=0) -> (element=w816:string)
            n386 = call-poly <instrlib>:"Open.vi"("error in (no error)"=w823, "Device Identifier"=w816, "Mercury Reference In"=w817) -> ("error out"=w839:errorcluster, "Mercury Reference Out"=w838:T47)  [unwired: 7 out]
            n387 = call-poly <instrlib>:"Configuration (Read).vi"("error in"=w839, "Mercury Reference In"=w838) -> ("error out"=w844:errorcluster, "LVL Device Settings"=→"LVL Device DetailSettings":T23, "Mercury Reference Out"=w841:T47)  [unwired: 1 in, 6 out]
            n388 = call-poly <instrlib>:"Configuration (Read).vi"("error in"=w844, "Mercury Reference In"=w841) -> ("error out"=w845:errorcluster, "Serial Number"=→"LVL S/N":string, "Mercury Reference Out"=w843:T47)  [unwired: 1 in, 6 out]
            n389 = call-poly <instrlib>:"Configuration (Read).vi"("error in"=w845, "Mercury Reference In"=w843) -> ("error out"=w848:errorcluster, "Resistance Configuration"=→"He Res Config":T28, "Mercury Reference Out"=w847:T47)  [unwired: 1 in, 6 out]
            n390 = call-poly <instrlib>:"Configuration (Read).vi"("error in"=w848, "Mercury Reference In"=w847) -> ("error out"=w850:errorcluster, "Magnitude"=→"LVL P Magnitude":dbl, "Mercury Reference Out"=w849:T47)  [unwired: 1 in, 6 out]
            n391 = call-poly <instrlib>:"Configuration (Read).vi"("error in"=w850, "Mercury Reference In"=w849) -> ("error out"=w822:errorcluster, "Duration"=→"LVL P Duration":dbl, "Mercury Reference Out"=w820:T47)  [unwired: 1 in, 6 out]
            n392 = call-poly <instrlib>:"Configuration (Read).vi"("error in"=w822, "Mercury Reference In"=w820) -> ("error out"=w826:errorcluster, "Freq 100%"=→"N Freq 100%":dbl, "Mercury Reference Out"=w825:T47)  [unwired: 1 in, 6 out]
            n393 = call-poly <instrlib>:"Configuration (Read).vi"("error in"=w826, "Mercury Reference In"=w825) -> ("error out"=w829:errorcluster, "Pulse Period"=→"N Pulse Period":dbl, "Mercury Reference Out"=w828:T47)  [unwired: 1 in, 6 out]
            n394 = call-poly <instrlib>:"Signals (Read).vi"("error in"=w829, "Mercury Reference In"=w828) -> ("error out"=w831:errorcluster, "Resistance"=→"He Resistance":dbl, "Mercury Reference Out"=w830:T47)  [unwired: 1 in, 6 out]
            n395 = call-poly <instrlib>:"Signals (Read).vi"("error in"=w831, "Mercury Reference In"=w830) -> ("error out"=w833:errorcluster, "Level"=→"He Level" →"He LEVEL":dbl, "Mercury Reference Out"=w832:T47)  [unwired: 1 in, 6 out]
            n396 = call-poly <instrlib>:"Signals (Read).vi"("error in"=w833, "Mercury Reference In"=w832) -> ("error out"=w835:errorcluster, "Counter"=→"N Counter":u32, "Mercury Reference Out"=w834:T47)  [unwired: 1 in, 6 out]
            n397 = call-poly <instrlib>:"Signals (Read).vi"("error in"=w835, "Mercury Reference In"=w834) -> ("error out"=w821:errorcluster, "Level"=→"N Level" →"N2 LEVEL":dbl)  [unwired: 1 in, 7 out]
            n398 = call <vilib>:"Add State(s) to Queue__jki_lib_state_machine.vi"("State(s) in (\"\")"=w855) -> ("States Out"=w856:string)  [unwired: 14 in]
          }
          frame "Mercury: Query IPS: Temperature" {
            n399 = Unbundle By Name(w901) -> ("Mercury IPS Ref"=w858:T47)
            n400 = local read "IPS Devices"() -> (w900:string[])
            n401 = Index Array(array=w900, index=4) -> (element=w859:string)
            n402 = call-poly <instrlib>:"Open.vi"("error in (no error)"=w857, "Device Identifier"=w859, "Mercury Reference In"=w858) -> ("error out"=w888:errorcluster, "Mercury Reference Out"=w883:T47)  [unwired: 7 out]
            n403 = call-poly <instrlib>:"Configuration (Read).vi"("error in"=w888, "Mercury Reference In"=w883) -> ("error out"=w889:errorcluster, "Serial Number"=→"Temp S/N 2":string, "Mercury Reference Out"=w884:T47)  [unwired: 1 in, 6 out]
            n404 = call-poly <instrlib>:"Configuration (Read).vi"("error in"=w889, "Mercury Reference In"=w884) -> ("error out"=w890:errorcluster, "Nickname"=→"T Nickname 2":string, "Mercury Reference Out"=w885:T47)  [unwired: 1 in, 6 out]
            n405 = call-poly <instrlib>:"Configuration (Read).vi"("error in"=w890, "Mercury Reference In"=w885) -> ("error out"=w891:errorcluster, "Unit"=→"Unit 12":T3, "Excitation Magnitude"=→"Excitation Magnitude 2":dbl, "Mercury Reference Out"=w886:T47)  [unwired: 1 in, 5 out]
            n406 = call-poly <instrlib>:"Configuration (Read).vi"("error in"=w891, "Mercury Reference In"=w886) -> ("error out"=w892:errorcluster, "Sensor Type"=→"Sensor Type 2":T6, "Mercury Reference Out"=w887:T47)  [unwired: 1 in, 6 out]
            n407 = call-poly <instrlib>:"Configuration (Read).vi"("error in"=w892, "Mercury Reference In"=w887) -> ("error out"=w862:errorcluster, "Excitation Type"=→"Excitation Type 2":T8, "Mercury Reference Out"=w861:T47)  [unwired: 1 in, 6 out]
            n408 = call-poly <instrlib>:"Configuration (Read).vi"("error in"=w862, "Mercury Reference In"=w861) -> ("error out"=w868:errorcluster, "Unit"=→"H Unit 2":T3, "Hot Limit"=→"Hot Limit 2":dbl, "Mercury Reference Out"=w863:T47)  [unwired: 1 in, 5 out]
            n409 = call-poly <instrlib>:"Configuration (Read).vi"("error in"=w868, "Mercury Reference In"=w863) -> ("error out"=w869:errorcluster, "Unit"=→"C Unit 2":T3, "Cold Limit"=→"Cold Limit 2":dbl, "Mercury Reference Out"=w864:T47)  [unwired: 1 in, 5 out]
            n410 = call-poly <instrlib>:"Signals (Read).vi"("error in"=w869, "Mercury Reference In"=w864) -> ("error out"=w870:errorcluster, "Unit"=→"V Unit 2":T3, "Voltage"=→"Voltage 2":dbl, "Mercury Reference Out"=w865:T47)  [unwired: 1 in, 5 out]
            n411 = call-poly <instrlib>:"Signals (Read).vi"("error in"=w870, "Mercury Reference In"=w865) -> ("error out"=w871:errorcluster, "Unit"=→"T Unit 2":T3, "Temperature"=→"Temperature 2":dbl, "Mercury Reference Out"=w866:T47)  [unwired: 1 in, 5 out]
            n412 = call-poly <instrlib>:"Configuration (Read).vi"("error in"=w871, "Mercury Reference In"=w866) -> ("error out"=w872:errorcluster, "Device Details"=→"Temperature Device Settings 2":T4, "Mercury Reference Out"=w867:T47)  [unwired: 1 in, 6 out]
            n413 = call-poly <instrlib>:"Configuration (Read).vi"("error in"=w872, "Mercury Reference In"=w867) -> ("error out"=w860:errorcluster, "Loop Details"=→"T Loop Details 2":T11)  [unwired: 1 in, 7 out]
            n414 = call <vilib>:"Add State(s) to Queue__jki_lib_state_machine.vi"("State(s) in (\"\")"=w902) -> ("States Out"=w903:string)  [unwired: 14 in]
          }
          frame "Mercury: Query IPS: Magnet" {
            n415 = Unbundle By Name(w942) -> ("Mercury IPS Ref"=w908:T47)
            n416 = call-poly <instrlib>:"Open.vi"("error in (no error)"=w904, "Device Identifier"="Device Identifier", "Mercury Reference In"=w908) -> ("error out"=w927:errorcluster, "Mercury Reference Out"=w926:T47)  [unwired: 7 out]
            n417 = call-poly <instrlib>:"Configuration (Read).vi"("error in"=w927, "Mercury Reference In"=w926) -> ("error out"=w930:errorcluster, "Magnet Device Details"=→"Magnet Device Details":T31, "Mercury Reference Out"=w929:T47)  [unwired: 1 in, 6 out]
            n418 = call-poly <instrlib>:"Configuration (Read).vi"("error in"=w930, "Mercury Reference In"=w929) -> ("error out"=w933:errorcluster, "Serial Number"=→"Mag S/N":string, "Mercury Reference Out"=w932:T47)  [unwired: 1 in, 6 out]
            n419 = call-poly <instrlib>:"Configuration (Read).vi"("error in"=w933, "Mercury Reference In"=w932) -> ("error out"=w936:errorcluster, "Bipolar Output"=→"Bipolar Output":string, "Mercury Reference Out"=w935:T47)  [unwired: 1 in, 6 out]
            n420 = call-poly <instrlib>:"Configuration (Read).vi"("error in"=w936, "Mercury Reference In"=w935) -> ("error out"=w939:errorcluster, "Out Config"=→"Out Config":T56, "Mercury Reference Out"=w938:T47)  [unwired: 1 in, 6 out]
            n421 = call-poly <instrlib>:"Configuration (Read).vi"("error in"=w939, "Mercury Reference In"=w938) -> ("error out"=w910:errorcluster, "Unit"=→"Unit 8":T3, "Current Limit"=→"Current Limit":dbl, "Mercury Reference Out"=w907:T47)  [unwired: 1 in, 5 out]
            n422 = call-poly <instrlib>:"Configuration (Read).vi"("error in"=w910, "Mercury Reference In"=w907) -> ("error out"=w913:errorcluster, "Unit"=→"Unit 9":T3, "AtoB"=→"AtoB":dbl, "Mercury Reference Out"=w912:T47)  [unwired: 1 in, 5 out]
            n423 = call-poly <instrlib>:"Configuration (Read).vi"("error in"=w913, "Mercury Reference In"=w912) -> ("error out"=w916:errorcluster, "Switch Present"=→"Switch Present":string, "Mercury Reference Out"=w915:T47)  [unwired: 1 in, 6 out]
            n424 = call-poly <instrlib>:"Configuration (Read).vi"("error in"=w916, "Mercury Reference In"=w915) -> ("error out"=w921:errorcluster, "Unit"=→"Unit 10":T3, "SW VLIM"=→"SW VLIM":dbl, "Mercury Reference Out"=w920:T47)  [unwired: 1 in, 5 out]
            n425 = call-poly <instrlib>:"Signals (Read).vi"("error in"=w921, "Mercury Reference In"=w920) -> ("error out"=w923:errorcluster, "Unit"=→"Unit 11":T3, "Current Rate"=→"Current Rate":dbl, "Mercury Reference Out"=w922:T47)  [unwired: 1 in, 5 out]
            n426 = call-poly <instrlib>:"Signals (Read).vi"("error in"=w923, "Mercury Reference In"=w922) -> ("error out"=w909:errorcluster, "PSU Act Stat"=→"PSU Act Stat":T37)  [unwired: 1 in, 7 out]
            n427 = call <vilib>:"Add State(s) to Queue__jki_lib_state_machine.vi"("State(s) in (\"\")"=w943) -> ("States Out"=w944:string)  [unwired: 14 in]
          }
          frame "Mercury: IPS: Idle - 1" {
            n428 = Unbundle By Name(w985) -> ("Mercury IPS Ref"=w953:T47)
            n429 = local read "Device Identifier"() -> (w966:T33)
            n430 = call-poly <instrlib>:"Configuration (Read).vi"("error in"=w984, "Mercury Reference In"=w953) -> ("error out"=w973:errorcluster, "Time"=w977:string, "Mercury Reference Out"=w974:T47)  [unwired: 1 in, 6 out]
            n431 = local write "Time 2"(w977) -> ()
            n432 = call-poly <instrlib>:"Open.vi"("error in (no error)"=w973, "Device Identifier"=w966, "Mercury Reference In"=w974) -> ("error out"=w972:errorcluster, "Mercury Reference Out"=w971:T47)  [unwired: 7 out]
            n433 = call-poly <instrlib>:"Signals (Read).vi"("error in"=w972, "Mercury Reference In"=w971) -> ("error out"=w983:errorcluster, "Switch Heater Status"=w975:string, "Mercury Reference Out"=w980:T47)  [unwired: 1 in, 6 out]
            n434 = Equal?(x=w975, y="ON") -> (x = y?=w950:bool)
            "SWITCH HEATER" <- w950
            n435 = call-poly <instrlib>:"Signals (Read).vi"("error in"=w983, "Mercury Reference In"=w980) -> ("error out"=w982:errorcluster, "Current"=→"Current (A)" →"Current (A)":dbl, "Mercury Reference Out"=w979:T47)  [unwired: 1 in, 6 out]
            n436 = call-poly <instrlib>:"Signals (Read).vi"("error in"=w982, "Mercury Reference In"=w979) -> ("error out"=w965:errorcluster, "Voltage"=→"Voltage (V) 2" →"Voltage (V)":dbl, "Mercury Reference Out"=w964:T47)  [unwired: 1 in, 6 out]
            n437 = call-poly <instrlib>:"Signals (Read).vi"("error in"=w965, "Mercury Reference In"=w964) -> ("error out"=w967:errorcluster, "Field"=→"Power Supply Field (T)":dbl, "Mercury Reference Out"=w970:T47)  [unwired: 1 in, 6 out]
            n438 = call-poly <instrlib>:"Signals (Read).vi"("error in"=w967, "Mercury Reference In"=w970) -> ("error out"=w968:errorcluster, "Target Field Rate"=→"Target  Rate (T/min)":dbl, "Mercury Reference Out"=w969:T47)  [unwired: 1 in, 6 out]
            n439 = call-poly <instrlib>:"Signals (Read).vi"("error in"=w968, "Mercury Reference In"=w969) -> ("error out"=w963:errorcluster, "Target Field"=→"Target Field (T)":dbl, "Mercury Reference Out"=w962:T47)  [unwired: 1 in, 6 out]
            n440 = call-poly <instrlib>:"Signals (Read).vi"("error in"=w963, "Mercury Reference In"=w962) -> ("error out"=w981:errorcluster, "Persistant Field"=→"Magnet Field (T)" →"Magnet Field (T) 2":dbl, "Mercury Reference Out"=w978:T47)  [unwired: 1 in, 6 out]
            n441 = call-poly <instrlib>:"Signals (Read).vi"("error in"=w981, "Mercury Reference In"=w978) -> ("error out"=w947:errorcluster, "PSU Act Stat"=w954:T37)  [unwired: 1 in, 7 out]
            n442 = call <userlib>:"FGV_PSP - Mercury Status.vi"("error in"=w947, "Function"=enum16{"write", "read"}."read") -> ("error out"=w949:errorcluster, "Status"=w946:T57)  [unwired: 4 in]
            n443 = local write "PSU Act Stat"(w954) -> ()
            n444 = Bundle By Name(cluster=w946, "Switch"=w950) -> (w945:T57)
            n445 = case shown="\"CLMP\"" w954 {
              selector: w954 -> [w988 _ _ _ _]
              tunnel: [w988 "Holding" "Ramping to Setpoint" "Ramping to Zero" "Clamped"] -> w961
              frame Default {
              }
              frame "HOLD" {
              }
              frame "RTOS" {
              }
              frame "RTOZ" {
              }
              frame "CLMP" {
              }
            }
            "Magnet Status 3" <- w961
            n446 = call <userlib>:"FGV_PSP - Mercury Status.vi"("error in"=w949, "Function"=enum16{"write", "read"}."write", "Status"=w945) -> ("error out"=w948:errorcluster)  [unwired: 3 in, 1 out]
            n447 = call <vilib>:"Add State(s) to Queue__jki_lib_state_machine.vi"("State(s) in (\"\")"=w986) -> ("States Out"=w987:string)  [unwired: 14 in]
          }
          frame "Mercury: IPS: Idle - 2" {
            n448 = Unbundle By Name(w1045) -> ("Mercury IPS Ref"=w1013:T47)
            n449 = local read "IPS Devices"() -> (w1039:string[])
            n450 = Index Array(array=w1039, index=0) -> (element=w1038:string)
            n451 = call-poly <instrlib>:"Open.vi"("error in (no error)"=w1025, "Device Identifier"=w1038, "Mercury Reference In"=w1013) -> ("error out"=w1041:errorcluster, "Mercury Reference Out"=w1042:T47)  [unwired: 7 out]
            n452 = call-poly <instrlib>:"Signals (Read).vi"("error in"=w1041, "Mercury Reference In"=w1042) -> ("error out"=w1043:errorcluster, "Level"=w993:dbl, "Mercury Reference Out"=w1044:T47)  [unwired: 1 in, 6 out]
            "He LVL Chart" <- w993
            "He LEVEL 3" <- w993
            n453 = Greater?(x=w993, y=20.0) -> (0:w1022:bool)
            n454 = Greater?(x=w993, y=50.0) -> (0:w1023:bool)
            n455 = call-poly <instrlib>:"Signals (Read).vi"("error in"=w1043, "Mercury Reference In"=w1044) -> ("error out"=w1028:errorcluster, "Level"=w1014:dbl)  [unwired: 1 in, 7 out]
            "N2 LVL Chart" <- w1014
            n456 = case shown="False" w1022 {
              tunnel: [w1053 u32 6618880] -> w1011
              tunnel: w1023 -> [w1054 _]
              frame False {
                n457 = case shown="False" w1054 {
                  tunnel: [u32 16711680 u32 16776704] -> w1053
                  frame False {
                  }
                  frame True {
                  }
                }
              }
              frame True {
              }
            }
            n458 = local write "He LEVEL"(w993) -> ()
            n459 = local read "IPS Devices"() -> (w1033:string[])
            n460 = property on="He LVL Chart" class="Slide (strict)"("Fill Color"=w1011) -> ()  [unwired: 2 in, 2 out]
            n461 = property on="He LEVEL 3" class="DigNum (strict)"("NumText.TextColor"=w1011) -> ()  [unwired: 2 in, 2 out]
            n462 = local write "N2 LEVEL"(w1014) -> ()
            n463 = Index Array(array=w1033, index=5) -> (element=w1031:string)
            n464 = local read "Target  Rate (T/min)"() -> (w1003:dbl)
            n465 = local read "Power Supply Field (T)"() -> (w1001:dbl)
            n466 = call-poly <instrlib>:"Open.vi"("error in (no error)"=w1028, "Device Identifier"=w1031, "Mercury Reference In"=w1013) -> ("error out"=w1030:errorcluster, "Mercury Reference Out"=w1029:T47)  [unwired: 7 out]
            n467 = local read "Magnet Field (T) 2"() -> (w1000:dbl)
            n468 = Greater?(x=w1014, y=20.0) -> (0:w1016:bool)
            n469 = Greater?(x=w1014, y=50.0) -> (0:w1015:bool)
            n470 = local read "Target Field (T)"() -> (w1002:dbl)
            n471 = local read "Current (A)"() -> (w1005:dbl)
            n472 = local read "Voltage (V)"() -> (w1004:dbl)
            n473 = case shown="False" w1016 {
              tunnel: [w1048 u32 6618880] -> w1012
              tunnel: w1015 -> [w1049 _]
              frame False {
                n474 = case shown="False" w1049 {
                  tunnel: [u32 16711680 u32 16776704] -> w1048
                  frame False {
                  }
                  frame True {
                  }
                }
              }
              frame True {
              }
            }
            n475 = call-poly <instrlib>:"Signals (Read).vi"("error in"=w1030, "Mercury Reference In"=w1029) -> ("error out"=w998:errorcluster, "Temperature"=w995:dbl, "Mercury Reference Out"=w996:T47)  [unwired: 1 in, 6 out]
            "Magnet T" <- w995
            n476 = call-poly <instrlib>:"Signals (Read).vi"("error in"=w998, "Mercury Reference In"=w996) -> ("error out"=w997:errorcluster, "Resistance"=w994:dbl)  [unwired: 1 in, 7 out]
            "Magnet R" <- w994
            n477 = property on="N2 LVL Chart" class="Slide (strict)"("Fill Color"=w1012) -> ()  [unwired: 2 in, 2 out]
            n478 = property on="N2 LEVEL" class="DigNum (strict)"("NumText.TextColor"=w1012) -> ()  [unwired: 2 in, 2 out]
            n479 = local read "PSU Act Stat"() -> (w1021:string)
            n480 = call <userlib>:"FGV_PSP - Mercury Status.vi"("error in"=w997, "Function"=enum16{"write", "read"}."read") -> ("error out"=w1008:errorcluster, "Status"=w1006:T57)  [unwired: 4 in]
            n481 = Bundle By Name(cluster=w1006, "Magnet Field"=w1000, "PS Field"=w1001, "Target Field"=w1002, "Target Field Rate"=w1003, "Voltage"=w1004, "Current"=w1005) -> (w1007:T57)
            n482 = call <userlib>:"FGV_PSP - Mercury Status.vi"("error in"=w1008, "Function"=enum16{"write", "read"}."write", "Status"=w1007) -> ("error out"=w1026:errorcluster)  [unwired: 3 in, 1 out]
            n483 = Bundle(cluster=T44 {"Magnet Field"=0.0, "PS Field"=0.0, "Target Field"=0.0, "Target Field Rate"=0.0, "Voltage"=0.0, "Current"=0.0}, "Magnet Field"=w1000, "PS Field"=w1001, "Target Field"=w1002, "Target Field Rate"=w1003, "Voltage"=w1004, "Current"=w1005) -> (w1010:T44)
            n484 = call <userlib>:"FGV_PSP - Mercury Action Status.vi"("error in"=w1026, "Function"=enum16{"write", "read"}."write", "Mercury Status"=w1021) -> ("error out"=w1024:errorcluster)  [unwired: 3 in, 1 out]
            n485 = Cluster To Array(cluster=w1010) -> (array=w1035:dbl[])
            n486 = Build Array(w1021) -> (w1027:string[])
            n487 = Build Array (concatenate)(w1035, w1014, w993, w995, w994) -> (w1034:dbl[])
            n488 = call "1820_IPS_to_DSC.vi"("str"=w1027, "dbl"=w1034) -> ()  [unwired: 2 in]
            n489 = call <vilib>:"Add State(s) to Queue__jki_lib_state_machine.vi"("State(s) in (\"\")"=w1046) -> ("States Out"=w1047:string)  [unwired: 14 in]
          }
          frame "Mercury: ITC: Idle" {
            n490 = Unbundle By Name(w1087) -> ("Mercury ITC Ref"=w1068:T52)
            n491 = local read "ITC Devices"() -> (w1083:string[])
            n492 = Index Array(array=w1083, index=3) -> (element=w1082:string)
            n493 = call-poly <instrlib>:"Open.vi"("error in (no error)"=w1063, "Device Identifier"=w1082, "Mercury Reference In"=w1068) -> ("error out"=w1081:errorcluster, "Mercury Reference Out"=w1075:T47)  [unwired: 7 out]
            n494 = call-poly <instrlib>:"Signals (Read).vi"("error in"=w1081, "Mercury Reference In"=w1075) -> ("error out"=w1061:errorcluster, "Temperature"=w1066:dbl, "Mercury Reference Out"=w1060:T47)  [unwired: 1 in, 6 out]
            "LPF T" <- w1066
            n495 = call-poly <instrlib>:"Signals (Read).vi"("error in"=w1061, "Mercury Reference In"=w1060) -> ("error out"=w1059:errorcluster, "Resistance"=w1058:dbl)  [unwired: 1 in, 7 out]
            "LPF R" <- w1058
            n496 = local read "ITC Devices"() -> (w1086:string[])
            n497 = Index Array(array=w1086, index=1) -> (element=w1084:string)
            n498 = call-poly <instrlib>:"Open.vi"("error in (no error)"=w1059, "Device Identifier"=w1084, "Mercury Reference In"=w1068) -> ("error out"=w1080:errorcluster, "Mercury Reference Out"=w1079:T47)  [unwired: 7 out]
            n499 = call-poly <instrlib>:"Configuration (Read).vi"("error in"=w1080, "Mercury Reference In"=w1079) -> ("error out"=w1074:errorcluster, "Device Details"=w1078:T15)  [unwired: 1 in, 7 out]
            n500 = local read "ITC Devices"() -> (w1072:string[])
            n501 = Unbundle By Name(w1078) -> ("Pressure Signals.Pressure"=w1077:string)
            n502 = Index Array(array=w1072, index=0) -> (element=w1071:string)
            n503 = call-poly <instrlib>:"Open.vi"("error in (no error)"=w1074, "Device Identifier"=w1071, "Mercury Reference In"=w1068) -> ("error out"=w1070:errorcluster, "Mercury Reference Out"=w1069:T47)  [unwired: 7 out]
            n504 = Fract/Exp String To Number(string=w1077) -> (number=w1065:dbl)  [unwired: 3 in, 1 out]
            "LPF Pressure" <- w1065
            n505 = call-poly <instrlib>:"Signals (Read).vi"("error in"=w1070, "Mercury Reference In"=w1069) -> ("error out"=w1062:errorcluster, "% Open"=w1064:dbl)  [unwired: 1 in, 7 out]
            "LPF NV (%)" <- w1064
            n506 = Build Array(w1066, w1065, w1064, w1058) -> (w1067:dbl[])
            n507 = call "1820_ITC_to_DSC.vi"("dbl"=w1067) -> ()  [unwired: 3 in]
            n508 = call <vilib>:"Add State(s) to Queue__jki_lib_state_machine.vi"("State(s) in (\"\")"=w1088) -> ("States Out"=w1089:string)  [unwired: 14 in]
          }
          frame "Mercury: Empty" {
            n509 = Unbundle By Name(w1091) -> ()  [unwired: 1 out]
            n510 = call <vilib>:"Add State(s) to Queue__jki_lib_state_machine.vi"("State(s) in (\"\")"=w1092) -> ("States Out"=w1093:string)  [unwired: 14 in]
          }
          frame "Mercury: IPS: Idle - 3" {
            n511 = call "Oxford_MNK_Omega_Sign.vi"("error in (no error)"=w1095) -> ("error out"=w1094:errorcluster)  [unwired: 10 in]
            n512 = call <vilib>:"Add State(s) to Queue__jki_lib_state_machine.vi"("State(s) in (\"\")"=w1097) -> ("States Out"=w1098:string)  [unwired: 14 in]
          }
        }
      }
      n513 = disable-structure shown="Disabled" {
        frame Disabled {
          (unwired) FALSE
          n514 = call-poly <instrlib>:"Configuration (Read).vi"() -> ()  [unwired: 3 in, 9 out]
          n515 = disable-structure shown="Disabled" {
            frame Disabled {
              n516 = property on="Fast/Slow Fill" class="Bool (strict)" props=["Val(Sgnl)"]() -> ()  [unwired: 3 in, 2 out]
            }
            frame Enabled {
            }
          }
          n517 = local read "PS Heat"() -> ()  [unwired: 1 in]
          n518 = local read "Lambda"() -> ()  [unwired: 1 in]
          n519 = local write "PS Heat"(FALSE) -> ()
          n520 = local read "Clamp"() -> ()  [unwired: 1 out]
        }
        frame Enabled {
        }
      }
    }
    frame Enabled {
    }
  }
